vi "ScenarioScript.vi"(0 "Control In":T1) -> (1 "Control Out":T1, 2 "String":string)   [LabVIEW 2013]
uses:
  <vilib>/imath/engines/lvmath/Plug In/_Char/NIMS_CH_character datatype.ctl
  Global.vi
  <vilib>/imath/engines/lvmath2/RunTimeEngine/ErrorHandling/NIMS_Finalize Error.vi
  <vilib>/imath/engines/lvmath2/RunTimeEngine/Managers/WorkSpace/UID Generator.vi
  <vilib>/imath/engines/lvmath2/RunTimeEngine/RunTimeType/NIMS_RunTimeType_From StrictType (excl LVString).vi
  <instcachedir>/0/NIMS_RunTimeType_From StrictType (excl LVString)_4DEE718D6EB74582AA20236969C084FC.lvgen/NIMS_RunTimeType_From StrictType (excl LVString)_4DEE718D6EB74582AA20236969C084FC_033.vi
  <instcachedir>/0/NIMS_RunTimeType_From StrictType (excl LVString)_4DEE718D6EB74582AA20236969C084FC.lvgen/NIMS_RunTimeType_From StrictType (excl LVString)_4DEE718D6EB74582AA20236969C084FC_013.vi
  <instcachedir>/0/NIMS_RunTimeType_From StrictType (excl LVString)_4DEE718D6EB74582AA20236969C084FC.lvgen/NIMS_RunTimeType_From StrictType (excl LVString)_4DEE718D6EB74582AA20236969C084FC_010.vi
  <instcachedir>/0/NIMS_RunTimeType_From StrictType (excl LVString)_4DEE718D6EB74582AA20236969C084FC.lvgen/NIMS_RunTimeType_From StrictType (excl LVString)_4DEE718D6EB74582AA20236969C084FC_031.vi
  <instcachedir>/0/NIMS_RunTimeType_From StrictType (excl LVString)_4DEE718D6EB74582AA20236969C084FC.lvgen/NIMS_RunTimeType_From StrictType (excl LVString)_4DEE718D6EB74582AA20236969C084FC_008.vi
  <instcachedir>/0/NIMS_RunTimeType_From StrictType (excl LVString)_4DEE718D6EB74582AA20236969C084FC.lvgen/NIMS_RunTimeType_From StrictType (excl LVString)_4DEE718D6EB74582AA20236969C084FC_032.vi
  <vilib>/imath/engines/lvmath2/RunTimeEngine/Struct/NIMS_StructSetField.vi
  <vilib>/imath/engines/lvmath2/RunTimeEngine/Managers/SymbolTable/Clear UID.vi
  <vilib>/imath/engines/lvmath2/RunTimeEngine/Struct/NIMS_StructGetField.vi
  <vilib>/imath/engines/lvmath2/RunTimeEngine/RunTimeType/NIMS_RunTimeType_To Numeric.vi
  <instcachedir>/0/NIMS_RunTimeType_To Numeric_4795FB10E831402FABFA341B47E20681.lvgen/NIMS_RunTimeType_To Numeric_4795FB10E831402FABFA341B47E20681_011.vi
  <instcachedir>/0/NIMS_RunTimeType_To Numeric_4795FB10E831402FABFA341B47E20681.lvgen/NIMS_RunTimeType_To Numeric_4795FB10E831402FABFA341B47E20681_006.vi
  <instcachedir>/0/NIMS_RunTimeType_To Numeric_4795FB10E831402FABFA341B47E20681.lvgen/NIMS_RunTimeType_To Numeric_4795FB10E831402FABFA341B47E20681_004.vi
  <instcachedir>/0/NIMS_RunTimeType_To Numeric_4795FB10E831402FABFA341B47E20681.lvgen/NIMS_RunTimeType_To Numeric_4795FB10E831402FABFA341B47E20681_008.vi
  <instcachedir>/0/NIMS_RunTimeType_To Numeric_4795FB10E831402FABFA341B47E20681.lvgen/NIMS_RunTimeType_To Numeric_4795FB10E831402FABFA341B47E20681_010.vi
  <instcachedir>/0/NIMS_RunTimeType_To Numeric_4795FB10E831402FABFA341B47E20681.lvgen/NIMS_RunTimeType_To Numeric_4795FB10E831402FABFA341B47E20681_009.vi
  <vilib>/imath/engines/lvmath2/RunTimeEngine/NodeEndStatement/NIMS_NodeEndStatement_Output.vi
  <instcachedir>/0/NIMS_NodeEndStatement_Output_53EC0D466D134D7ABD903AC30B43404B.lvgen/NIMS_NodeEndStatement_Output_53EC0D466D134D7ABD903AC30B43404B_016.vi
  <instcachedir>/0/NIMS_NodeEndStatement_Output_53EC0D466D134D7ABD903AC30B43404B.lvgen/NIMS_NodeEndStatement_Output_53EC0D466D134D7ABD903AC30B43404B_015.vi
  <instcachedir>/0/NIMS_NodeEndStatement_Output_53EC0D466D134D7ABD903AC30B43404B.lvgen/NIMS_NodeEndStatement_Output_53EC0D466D134D7ABD903AC30B43404B_010.vi
  <vilib>/imath/engines/lvmath/Plug In/_Char/NIMS_CH_Character RV to String.vi
  <instcachedir>/0/NIMS_NodeEndStatement_Output_53EC0D466D134D7ABD903AC30B43404B.lvgen/NIMS_NodeEndStatement_Output_53EC0D466D134D7ABD903AC30B43404B_008.vi
  <instcachedir>/0/NIMS_RunTimeType_From StrictType (excl LVString)_4DEE718D6EB74582AA20236969C084FC.lvgen/NIMS_RunTimeType_From StrictType (excl LVString)_4DEE718D6EB74582AA20236969C084FC_009.vi
  <vilib>/imath/engines/lvmath2/RunTimeEngine/IndexRead/NIMS V(S).vi
  <instcachedir>/0/NIMS V(S)_0488751826AF41519A22953C041130DC.lvgen/NIMS V(S)_0488751826AF41519A22953C041130DC_000.vi
  <vilib>/imathl/engines/lvmath/Functions/Error Handling/Create Error.vi
  <vilib>/imath/engines/lvmath2/RunTimeEngine/BuiltInFunctions/sprintf/NIMS_sprintf(Str,RM).vi
  <vilib>/imath/engines/lvmath/Plug In/_Char/NIMS_CH_String to Character Array.vi
  <instcachedir>/0/NIMS_RunTimeType_From StrictType (excl LVString)_4DEE718D6EB74582AA20236969C084FC.lvgen/NIMS_RunTimeType_From StrictType (excl LVString)_4DEE718D6EB74582AA20236969C084FC_001.vi
  <vilib>/imath/engines/lvmath2/RunTimeEngine/LocalVariableDefStatement/MC_LocalVariableDefStatement_Display.vi
  <instcachedir>/0/NIMS V(S)_0488751826AF41519A22953C041130DC.lvgen/NIMS V(S)_0488751826AF41519A22953C041130DC_002.vi
  <instcachedir>/0/NIMS_RunTimeType_To Numeric_4795FB10E831402FABFA341B47E20681.lvgen/NIMS_RunTimeType_To Numeric_4795FB10E831402FABFA341B47E20681_003.vi
  <vilib>/imath/engines/lvmath2/RunTimeEngine/IndexReplace/NIMS V(S)=S.vi
  <instcachedir>/0/NIMS V(S)=S_66A18068148B4981A312229A93EA5C06.lvgen/NIMS V(S)=S_66A18068148B4981A312229A93EA5C06_000.vi
  <vilib>/imath/engines/lvmath2/RunTimeEngine/ErrorHandling/NIMS_Create Error From Enums.vi
  <instcachedir>/0/NIMS_NodeEndStatement_Output_53EC0D466D134D7ABD903AC30B43404B.lvgen/NIMS_NodeEndStatement_Output_53EC0D466D134D7ABD903AC30B43404B_001.vi
  <instcachedir>/0/NIMS V(S)_0488751826AF41519A22953C041130DC.lvgen/NIMS V(S)_0488751826AF41519A22953C041130DC_001.vi
  <vilib>/imath/engines/lvmath2/RunTimeEngine/IndexRead/NIMS M(S,S).vi
  <instcachedir>/0/NIMS M(S,S)_AC51E74150A542F7991B9634C66F3096.lvgen/NIMS M(S,S)_AC51E74150A542F7991B9634C66F3096_000.vi
  <instcachedir>/0/NIMS_NodeEndStatement_Output_53EC0D466D134D7ABD903AC30B43404B.lvgen/NIMS_NodeEndStatement_Output_53EC0D466D134D7ABD903AC30B43404B_011.vi
  <instcachedir>/0/NIMS V(S)=S_66A18068148B4981A312229A93EA5C06.lvgen/NIMS V(S)=S_66A18068148B4981A312229A93EA5C06_004.vi
  <vilib>/imath/engines/lvmath2/RunTimeEngine/BuiltInFunctions/abs/NIMS_abs(signed).vi
  <instcachedir>/0/NIMS_abs(signed)_C4FCB8E6058B49B797C7C8D53CA5F6EC.lvgen/NIMS_abs(signed)_C4FCB8E6058B49B797C7C8D53CA5F6EC_007.vi
  <instcachedir>/0/NIMS_RunTimeType_From StrictType (excl LVString)_4DEE718D6EB74582AA20236969C084FC.lvgen/NIMS_RunTimeType_From StrictType (excl LVString)_4DEE718D6EB74582AA20236969C084FC_000.vi
  <vilib>/imath/engines/lvmath2/RunTimeEngine/BuiltInFunctions/sprintf/NIMS_sprintf(Str,RS,RS).vi
  <vilib>/imath/engines/lvmath2/RunTimeEngine/BuiltInFunctions/length/NIMS_length(GV).vi
  <instcachedir>/0/NIMS_length(GV)_08A3D13377FD4E4B96F5795FBF3698FA.lvgen/NIMS_length(GV)_08A3D13377FD4E4B96F5795FBF3698FA_002.vi
  <vilib>/imath/engines/lvmath2/RunTimeEngine/BuiltInFunctions/zeros/NIMS_M=zeros(I32).vi
  <vilib>/imath/engines/lvmath2/RunTimeEngine/IndexReplace/NIMS M(S)=S.vi
  <instcachedir>/0/NIMS M(S)=S_4E994C4915F64874B0A495BA8935E304.lvgen/NIMS M(S)=S_4E994C4915F64874B0A495BA8935E304_001.vi
  <vilib>/imath/engines/lvmath2/RunTimeEngine/IndexRead/NIMS M(S).vi
  <instcachedir>/0/NIMS M(S)_B826C018497E4940AE96BD27B540B6FB.lvgen/NIMS M(S)_B826C018497E4940AE96BD27B540B6FB_000.vi
  <vilib>/imath/engines/lvmath2/RunTimeEngine/ArithmeticOperatorToken/NIMS_ArithmeticOperator_rightdiv.vi
  <instcachedir>/0/NIMS_ArithmeticOperator_rightdiv_C75411BD8BC84A93B6F1C8DA359A92EC.lvgen/NIMS_ArithmeticOperator_rightdiv_C75411BD8BC84A93B6F1C8DA359A92EC_000.vi
  <instcachedir>/0/NIMS V(S)=S_66A18068148B4981A312229A93EA5C06.lvgen/NIMS V(S)=S_66A18068148B4981A312229A93EA5C06_003.vi
  <vilib>/imath/engines/lvmath2/RunTimeEngine/CommandStatement/NIMS_CommandStatement_MaskErr.vi
  <vilib>/imath/engines/lvmath2/RunTimeEngine/BuiltInFunctions/sort/NIMS_[2o]_sort(RRowV,I32,Str).vi
  <instcachedir>/0/NIMS_[2o]_sort(RRowV,I32,Str)_CECB39279CEE49FE825BA66045B0C5B3.lvgen/NIMS_[2o]_sort(RRowV,I32,Str)_CECB39279CEE49FE825BA66045B0C5B3_000.vi
  <instcachedir>/0/NIMS_length(GV)_08A3D13377FD4E4B96F5795FBF3698FA.lvgen/NIMS_length(GV)_08A3D13377FD4E4B96F5795FBF3698FA_000.vi
  <vilib>/imath/engines/lvmath2/RunTimeEngine/CommandStatement/MC_CommandStatement_break.vi
  <vilib>/imath/engines/lvmath2/RunTimeEngine/BuiltInFunctions/findnz/NIMS_[1o]_findnz(GRowV).vi
  <instcachedir>/0/NIMS_[1o]_findnz(GRowV)_A907680C39E74AF18CBD76E991AC1137.lvgen/NIMS_[1o]_findnz(GRowV)_A907680C39E74AF18CBD76E991AC1137_001.vi
  <vilib>/imath/engines/lvmath2/RunTimeEngine/BuiltInFunctions/is_empty/NIMS_is_empty(GV).vi
  <instcachedir>/0/NIMS_is_empty(GV)_FC7E7C3D9544432CB6AA2416ADCF6D56.lvgen/NIMS_is_empty(GV)_FC7E7C3D9544432CB6AA2416ADCF6D56_000.vi
  <vilib>/imath/engines/lvmath2/RunTimeEngine/RowToken/NIMS_RowToken_M_SorRV.vi
  <instcachedir>/0/NIMS_RowToken_M_SorRV_6464340A296F47B6970F468C8541F43A.lvgen/NIMS_RowToken_M_SorRV_6464340A296F47B6970F468C8541F43A_001.vi
  <instcachedir>/0/NIMS M(S)_B826C018497E4940AE96BD27B540B6FB.lvgen/NIMS M(S)_B826C018497E4940AE96BD27B540B6FB_005.vi
  <vilib>/imath/engines/lvmath2/RunTimeEngine/BuiltInFunctions/rem/NIMS_rem_no checks.vi
  <instcachedir>/0/NIMS_rem_no checks_7935C26835844EFC868069820ED089DA.lvgen/NIMS_rem_no checks_7935C26835844EFC868069820ED089DA_008.vi
  <vilib>/imath/engines/lvmath2/RunTimeEngine/Managers/SymbolTable/NIMS_WorkSpace.lvlib
panel:
  out "SetMasterID":i32
  out "LapCounter":i32
  out "diference":dbl
  out "SlaveDistance":dbl
  out "MasterDistance":dbl
  out "Positioned":bool
  out "FirstTime":bool
  out "MasterID":i32
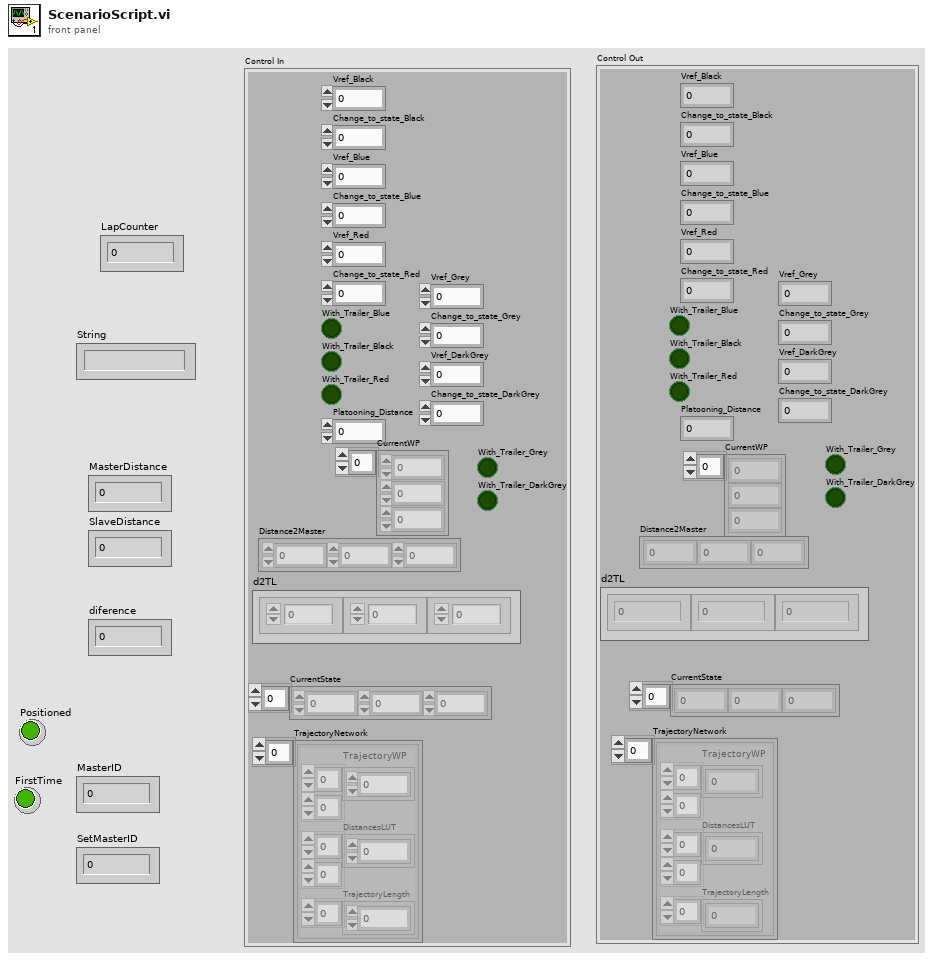
[diagram p1: front panel]
types:
  T1 = cluster{"Vref_Black":dbl, "Change_to_state_Black":i32, "Vref_Blue":dbl, "Change_to_state_Blue":i32, "Vref_Red":dbl, "Change_to_state_Red":i32, "Vref_Grey":dbl, "Change_to_state_Grey":i32, "Vref_DarkGrey":dbl, "Change_to_state_DarkGrey":i32, "With_Trailer_Blue":bool, "With_Trailer_Black":bool, "With_Trailer_Red":bool, "With_Trailer_Grey":bool, "With_Trailer_DarkGrey":bool, "Platooning_Distance":dbl, "CurrentWP":i32[], "Distance2Master":dbl[], "d2TL":dbl[], "CurrentState":i32[], "TrajectoryNetwork":cluster{"TrajectoryWP":dbl[][], "DistancesLUT":dbl[][], "TrajectoryLength":i32[]}[]}
  T2 = cluster{"TrajectoryWP":dbl[][], "DistancesLUT":dbl[][], "TrajectoryLength":i32[]}
  T3 = typedef "NIMS_CH_character datatype.ctl" = cluster{"Numeric":u8}
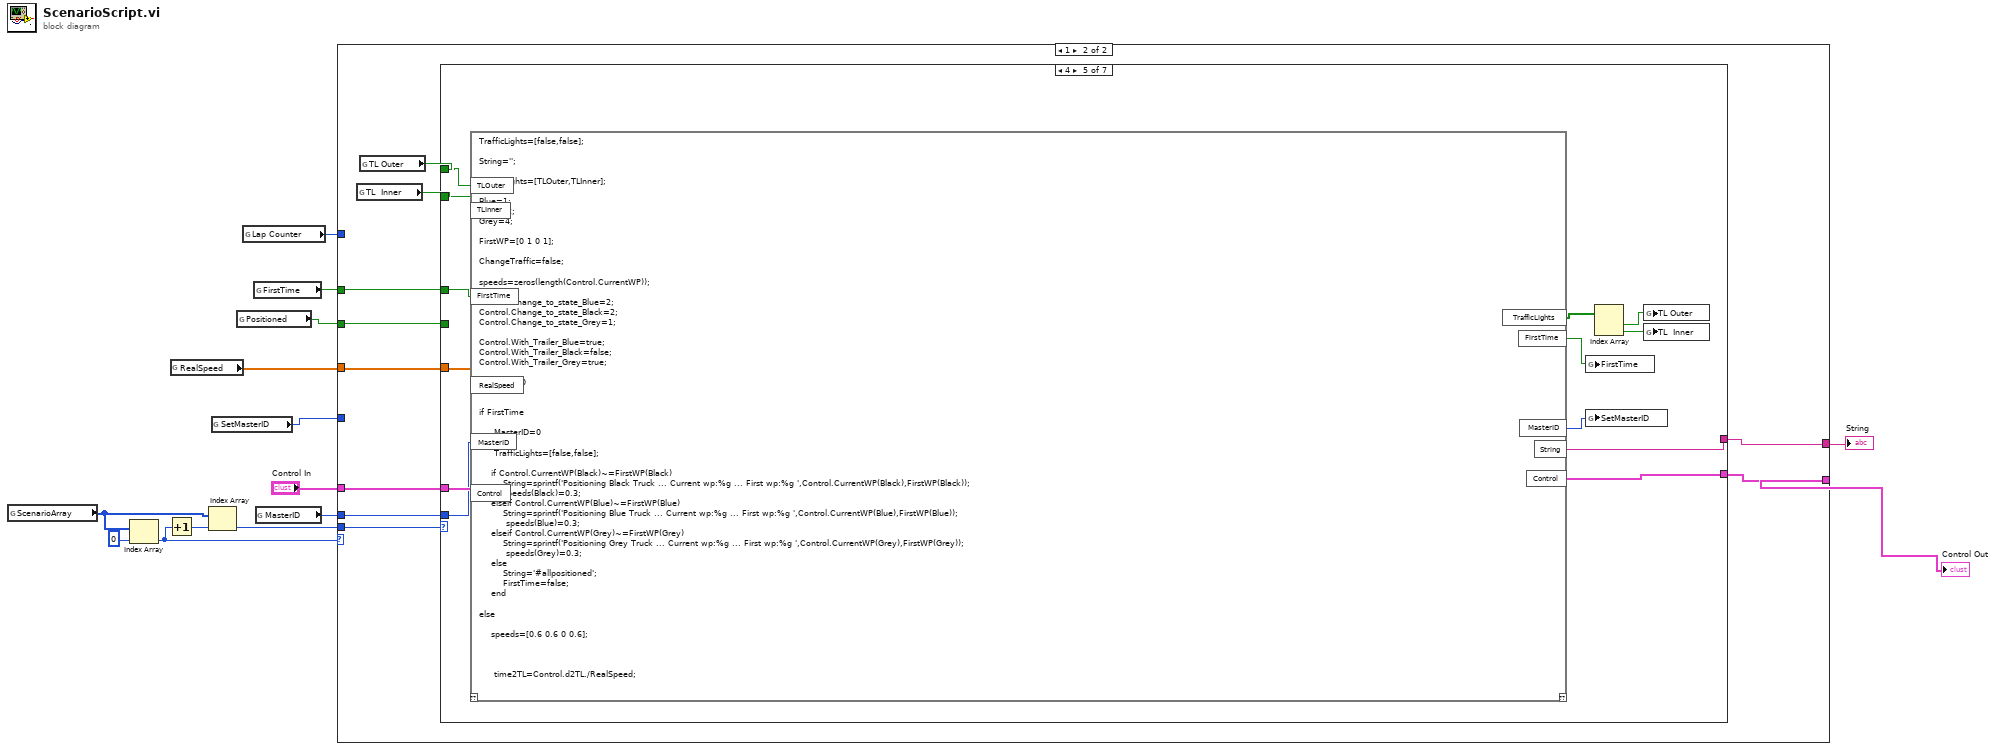
[diagram p0: block diagram]
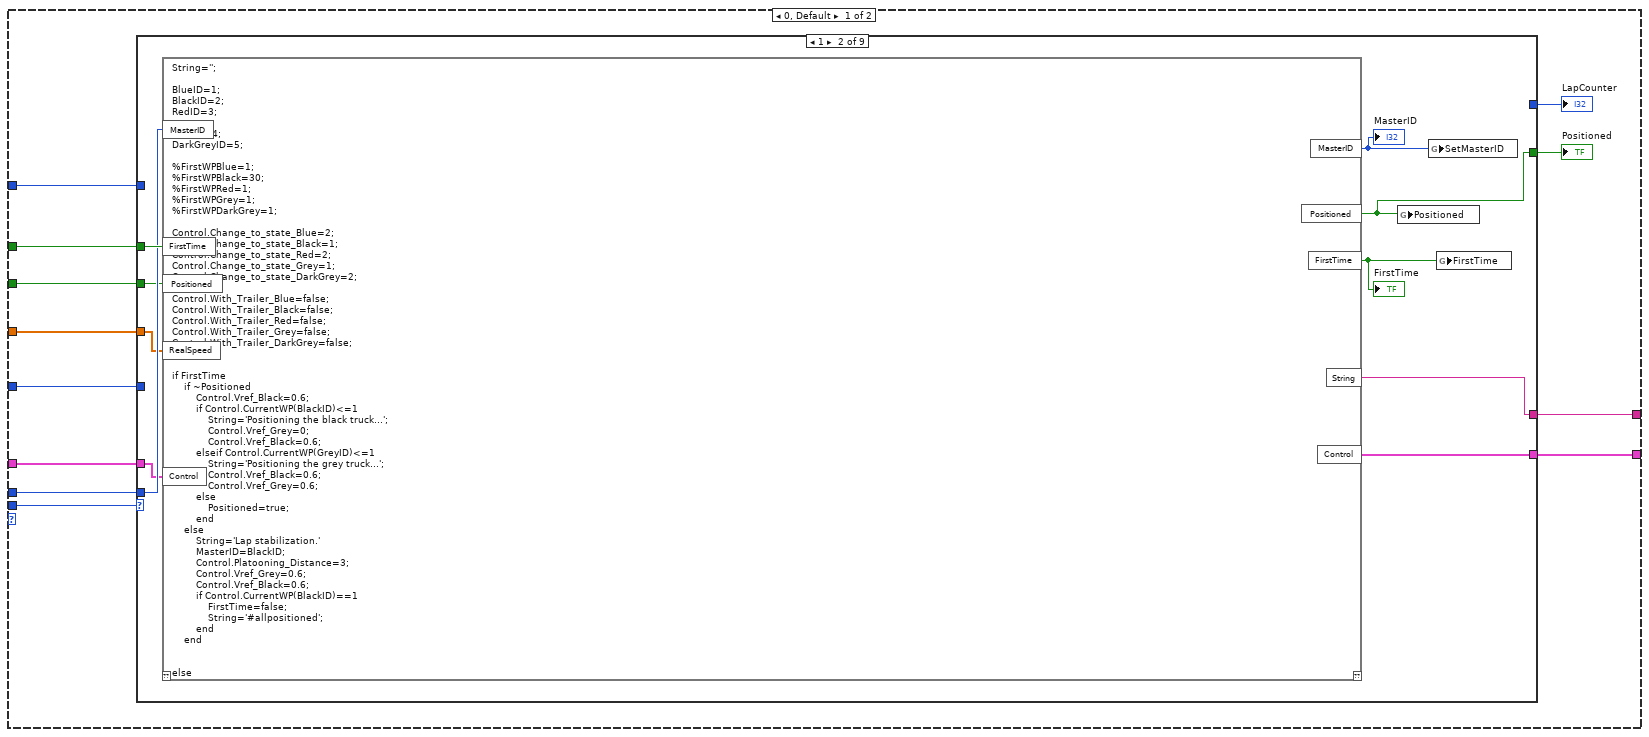
[diagram p2: hidden frame]
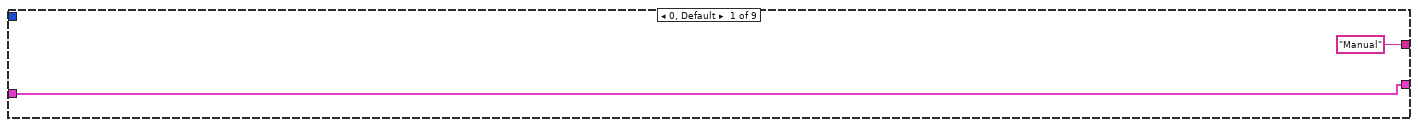
[diagram p3: hidden frame]
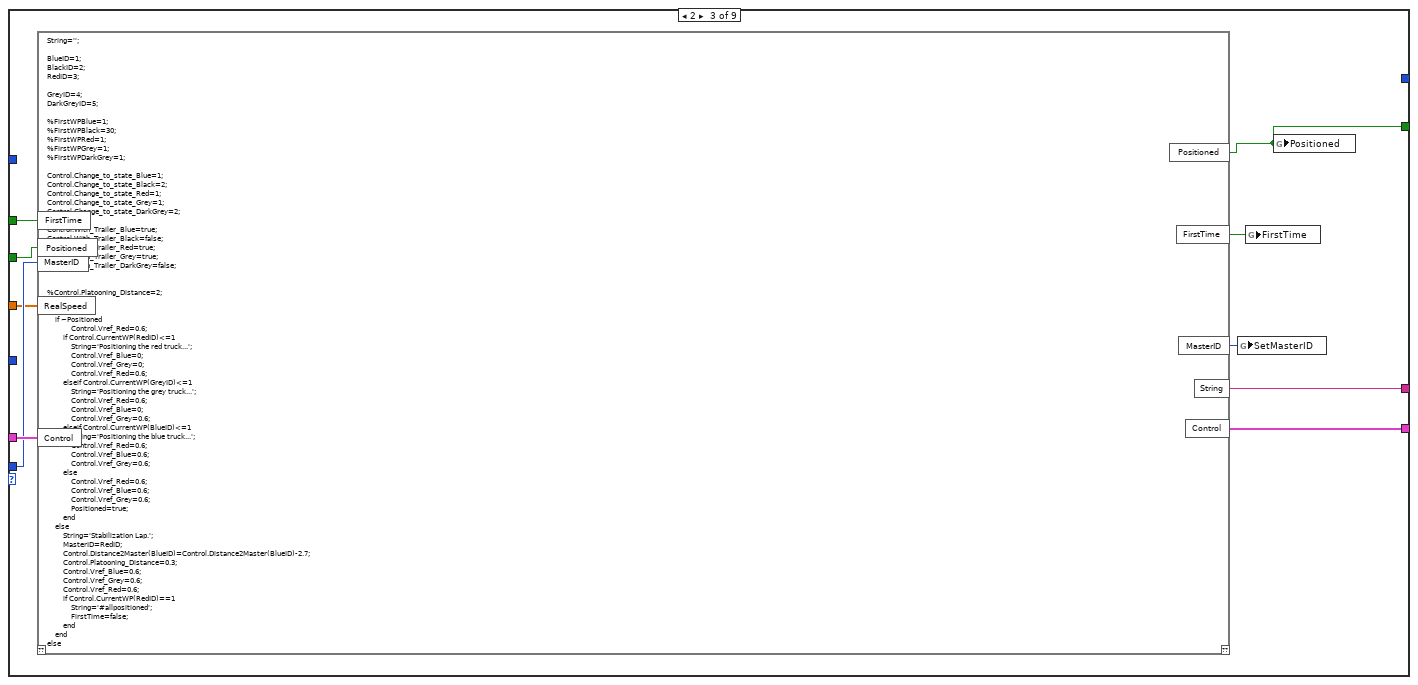
[diagram p4: hidden frame]
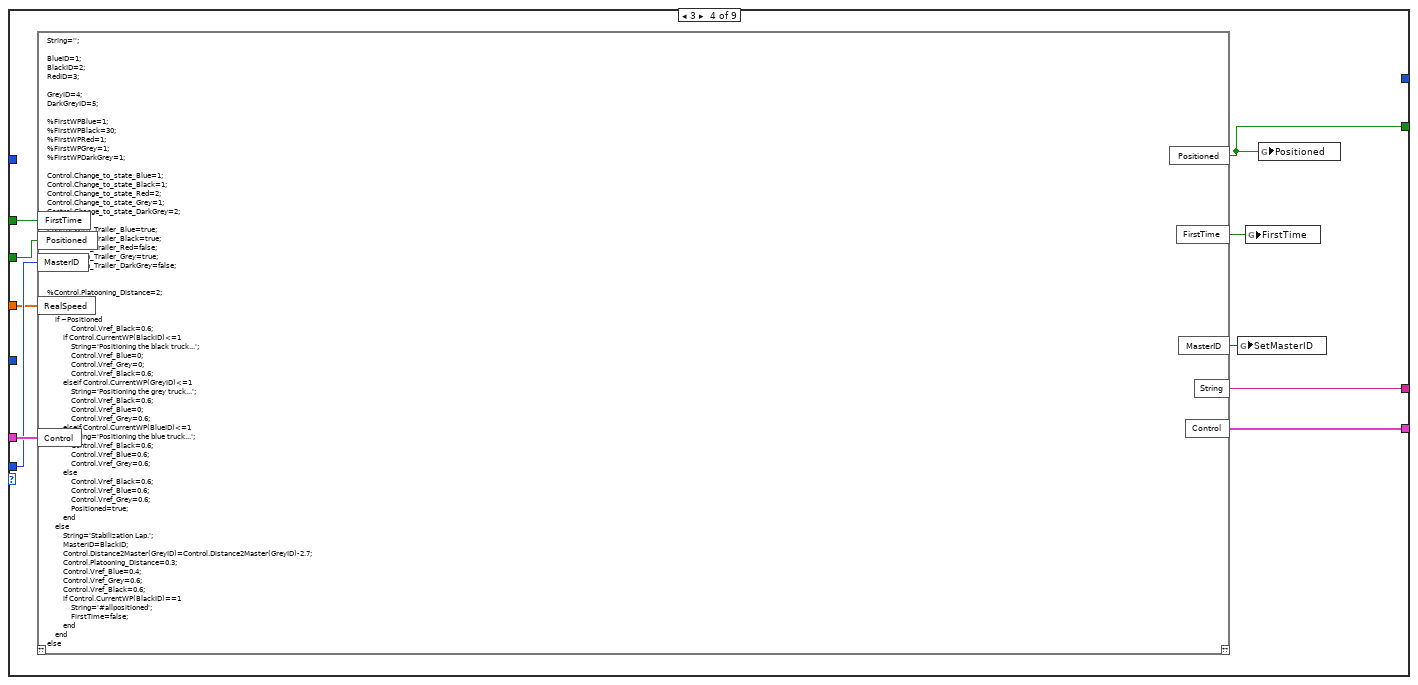
[diagram p5: hidden frame]
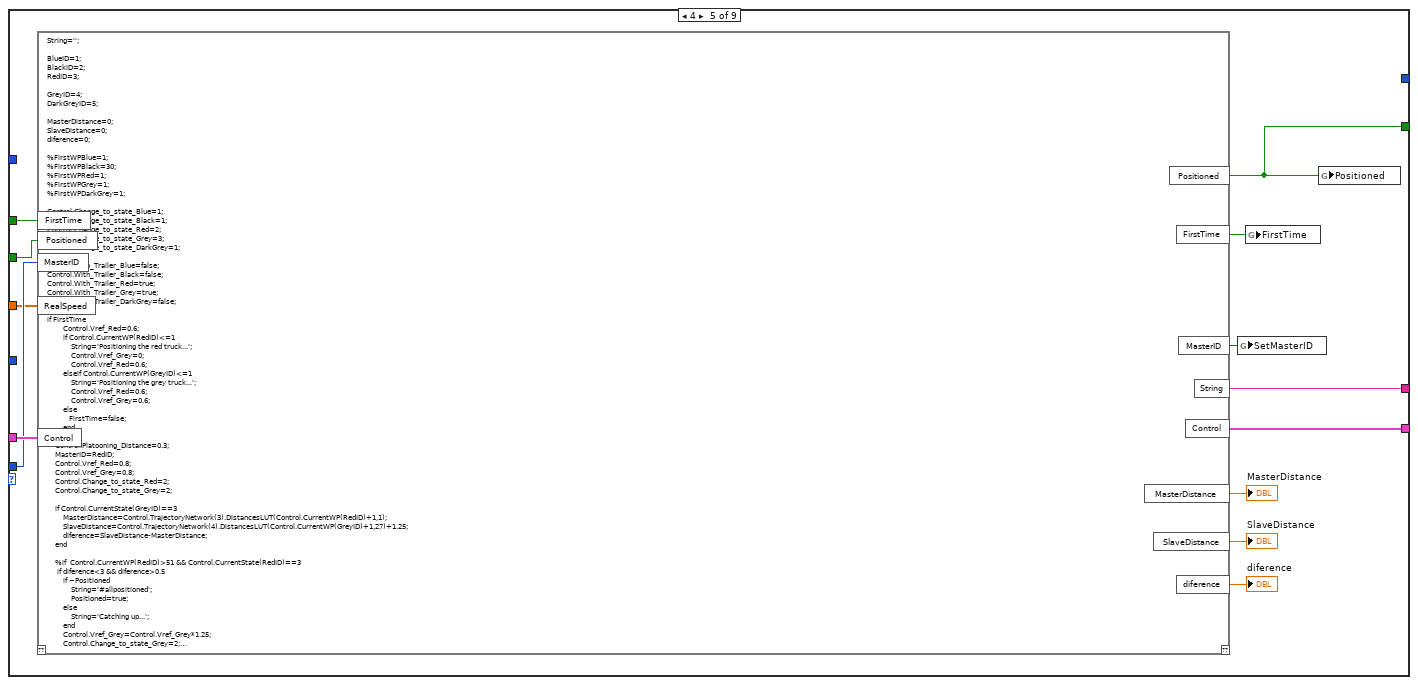
[diagram p6: hidden frame]
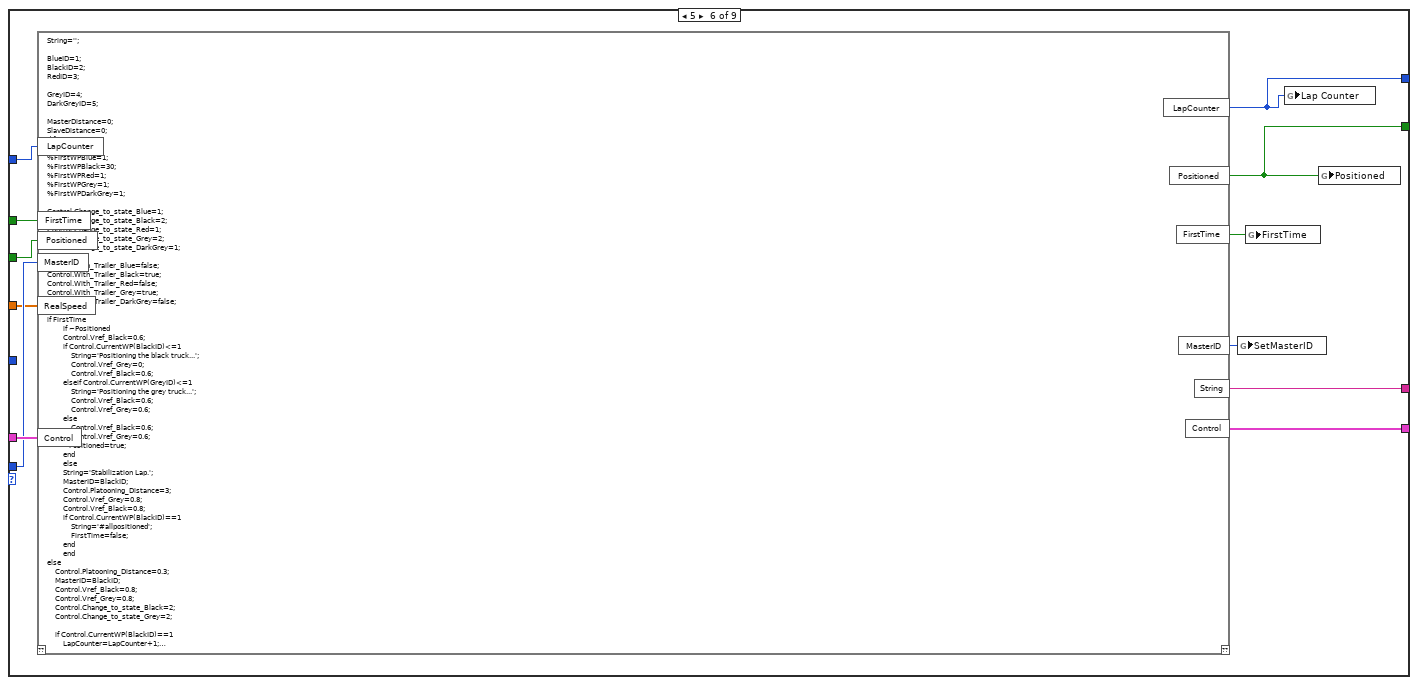
[diagram p7: hidden frame]
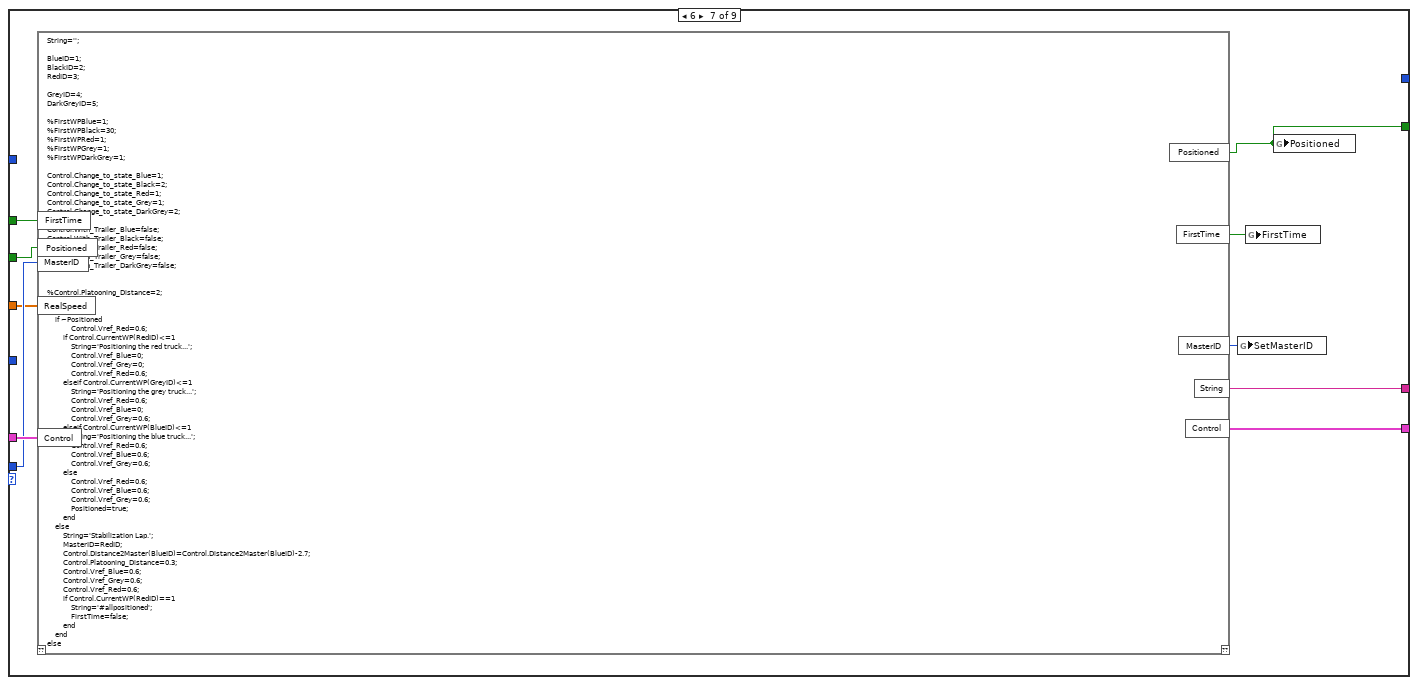
[diagram p8: hidden frame]
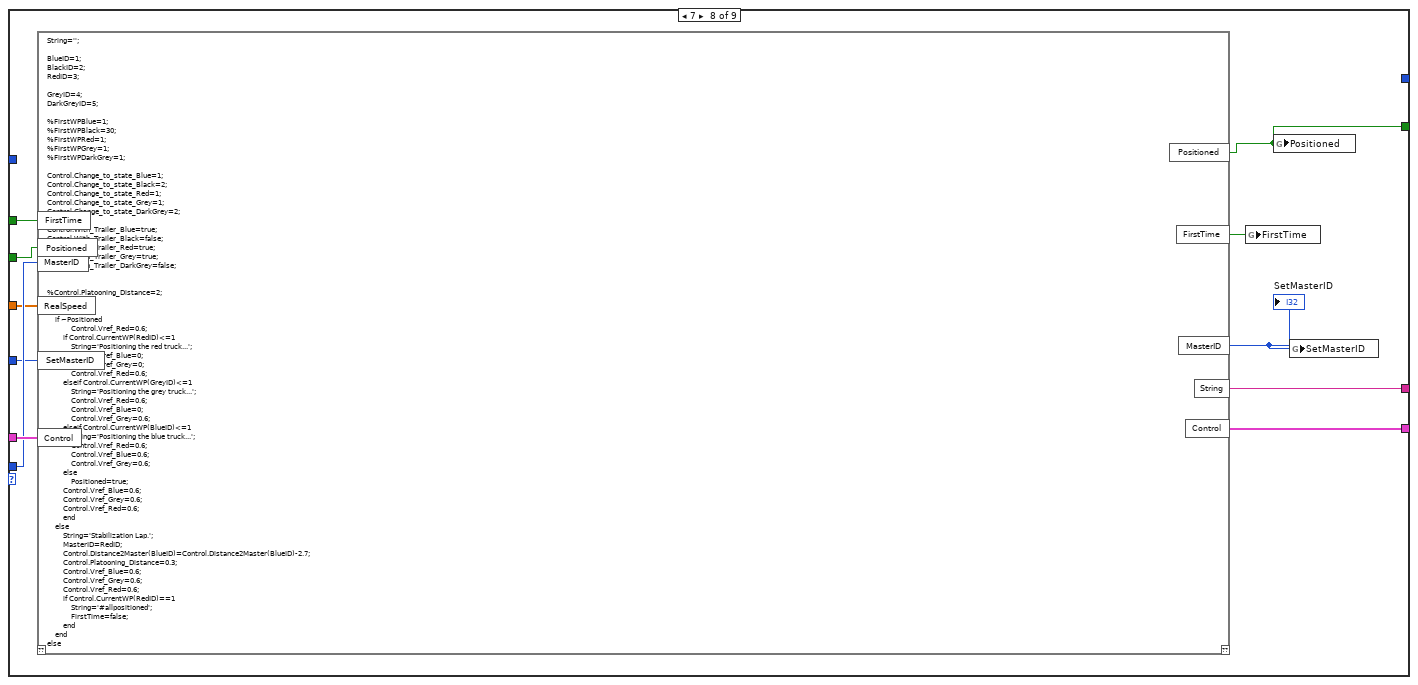
[diagram p9: hidden frame]
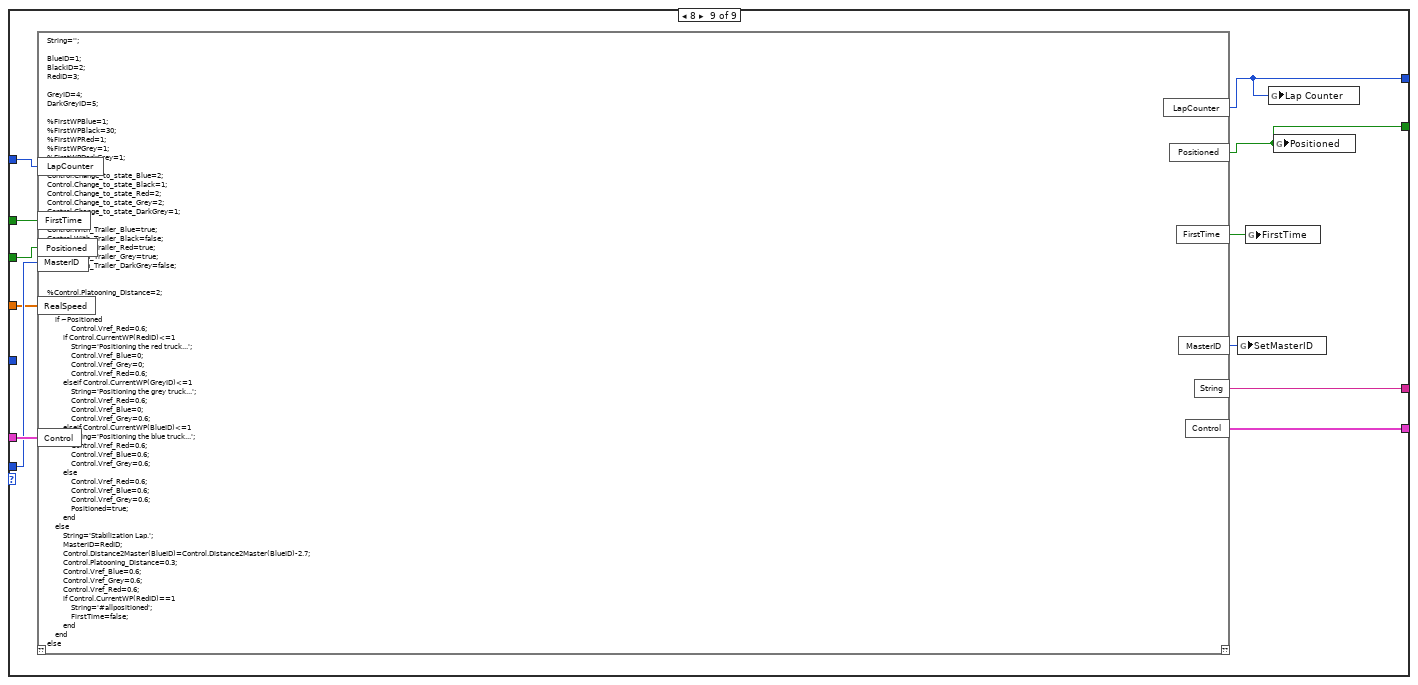
[diagram p10: hidden frame]
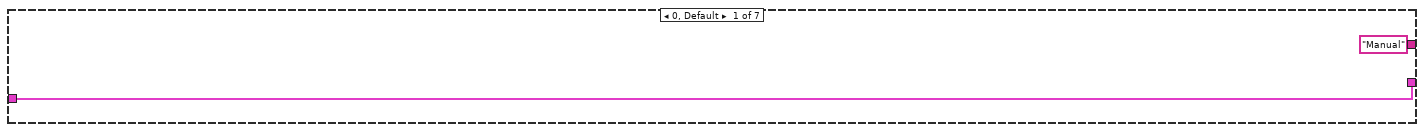
[diagram p11: hidden frame]
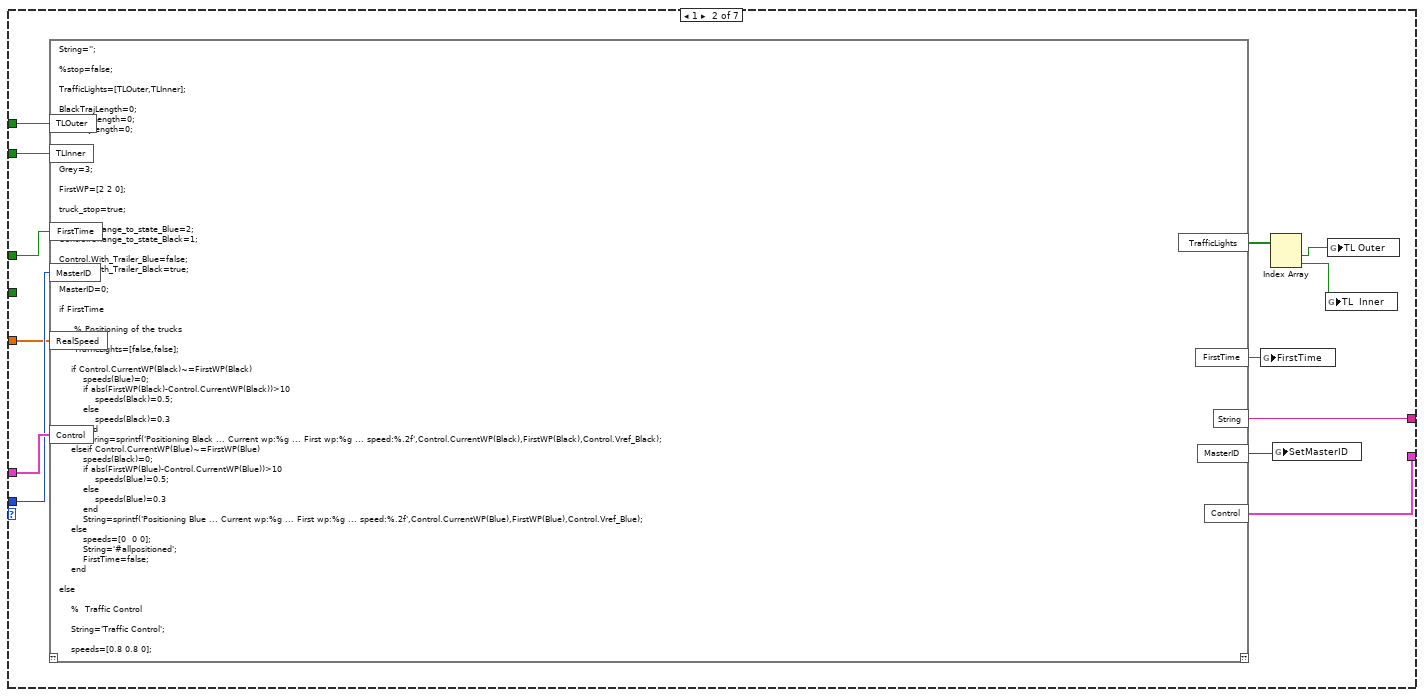
[diagram p12: hidden frame]
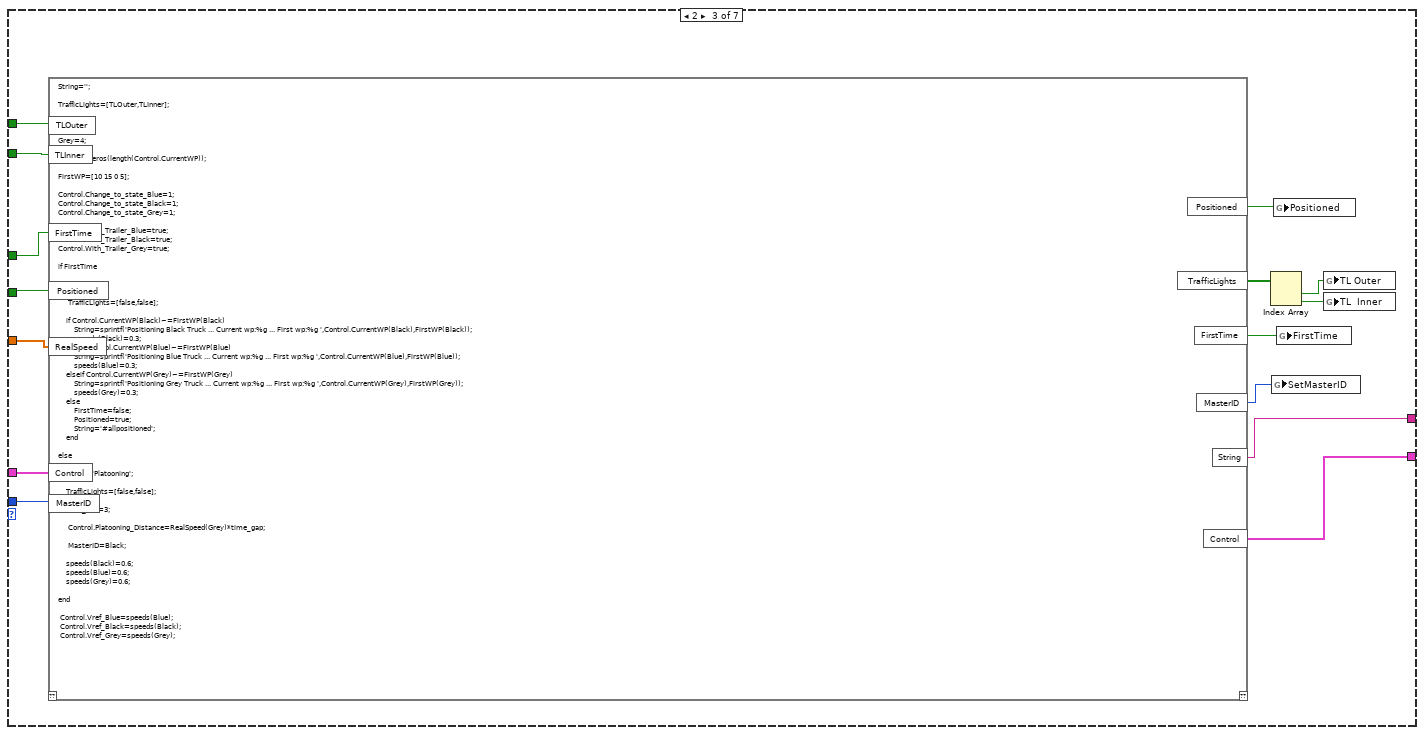
[diagram p13: hidden frame]
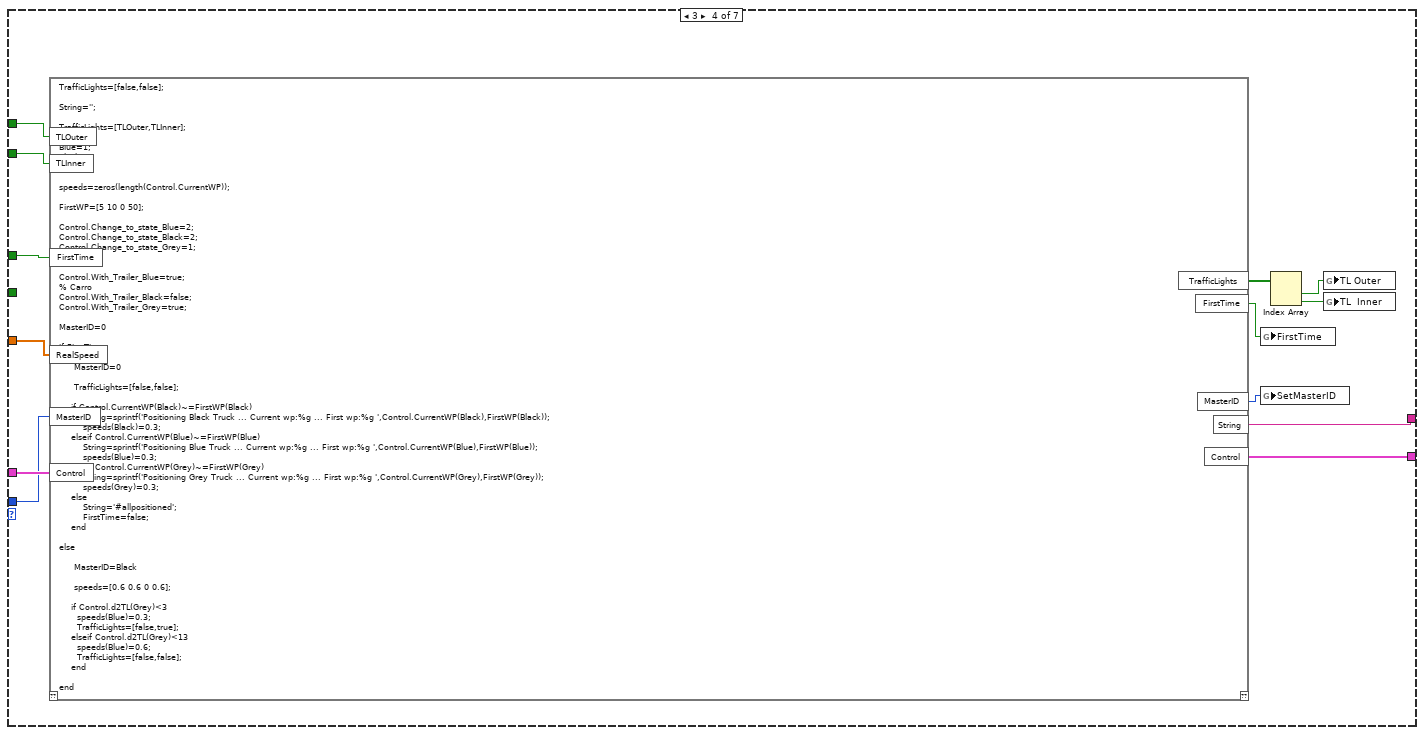
[diagram p14: hidden frame]
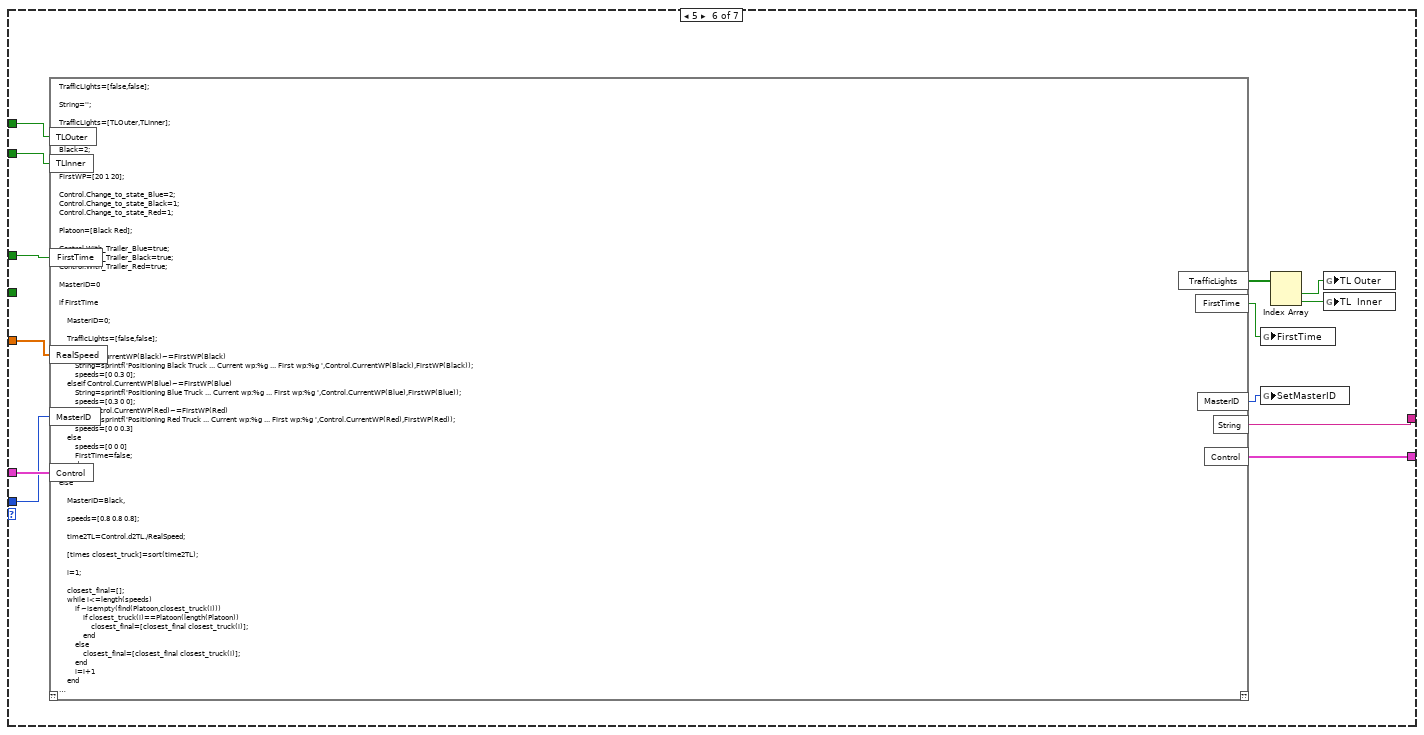
[diagram p15: hidden frame]
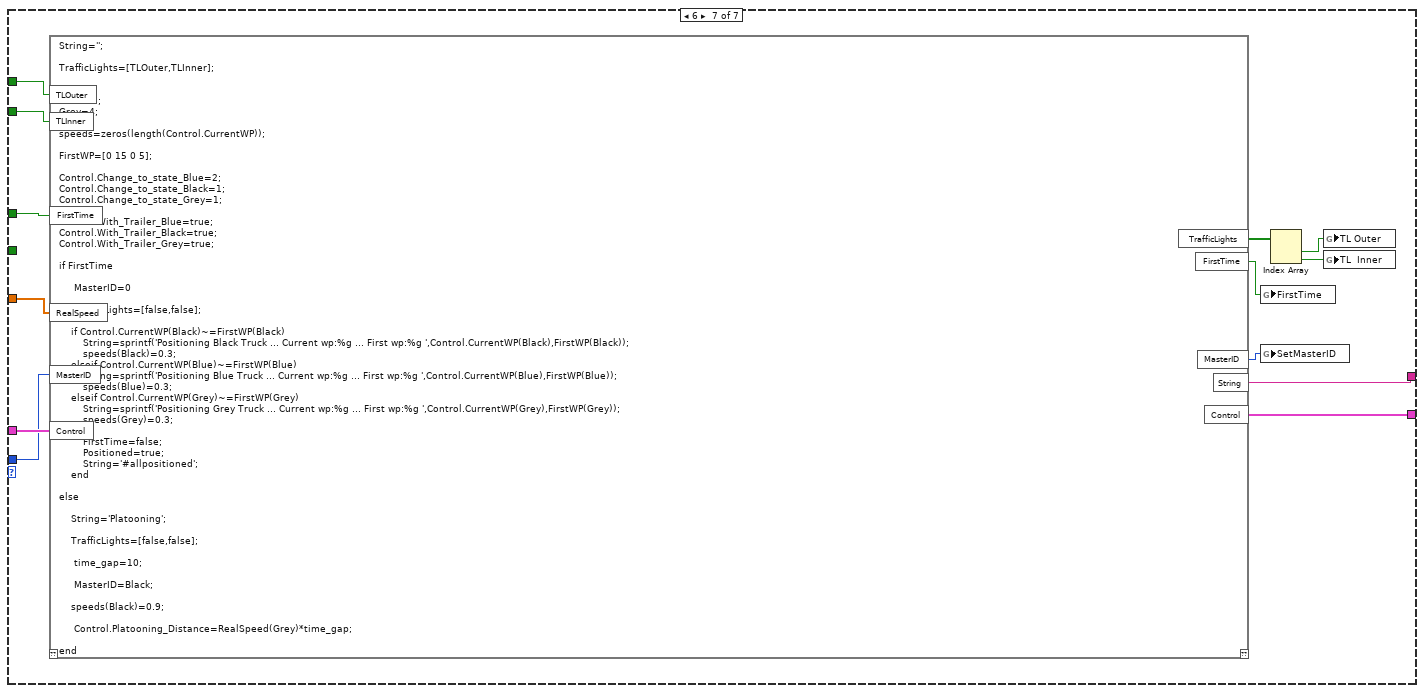
[diagram p16: hidden frame]
diagram:
  n1 = global read "Global.vi" "ScenarioArray"() -> (w13:u32[])
  n2 = Index Array(array=w13, index=0) -> (element=w12:u32)
  n3 = Increment(x=w12) -> (x+1=w11:u32)
  n4 = global read "Global.vi" "RealSpeed"() -> (w7:dbl[])
  n5 = Index Array(array=w13, index=w11) -> (element=w10:u32)
  n6 = global read "Global.vi" "SetMasterID"() -> (w1:i32)
  n7 = global read "Global.vi" "Positioned"() -> (w4:bool)
  n8 = global read "Global.vi" "Lap Counter"() -> (w2:i32)
  n9 = global read "Global.vi" "FirstTime"() -> (w9:bool)
  n10 = global read "Global.vi" "MasterID"() -> (w8:i32)
  n11 = case shown="1" w12 {
    tunnel: w10 -> [w26 w9910]
    tunnel: [w25 w9909] -> w3
    tunnel: w9 -> [w24 w9908]
    tunnel: w8 -> [w23 w9906]
    tunnel: w7 -> [w22 w9905]
    tunnel: "Control In" -> [w21 w9907]
    tunnel: [w20 w9902] -> w5
    tunnel: w4 -> [w19 w9901]
    tunnel: w2 -> [w17 _]
    tunnel: w1 -> [w15 _]
    frame 0, Default {
      n12 = case shown="1" w26 {
        tunnel: [w28 w38 w864 w2135 w3409 w4553 w5568 w6840 w8538] -> w25
        tunnel: w24 -> [_ w37 w861 w2132 w3406 w4550 w5565 w6837 w8535]
        tunnel: w23 -> [_ w35 w860 w2131 w3405 w4549 w5564 w6836 w8534]
        tunnel: w22 -> [_ w33 w859 w2130 w3404 w4548 w5563 w6835 w8533]
        tunnel: w21 -> [w28 w32 w862 w2133 w3407 w4551 w5566 w6838 w8536]
        tunnel: ["Manual" ("String") w31 w857 w2128 w3402 w4546 w5561 w6833 w8531] -> w20
        tunnel: w19 -> [_ w30 w856 w2127 w3401 w4545 w5560 w6832 w8530]
        tunnel: [_ w29 w855 w2126 w3400 w4544 w5559 w6831 w8529] -> w18
        tunnel: w17 -> [_ _ _ _ _ w4543 _ _ w8528]
        tunnel: [_ _ _ _ _ w4542 _ _ w8527] -> w16
        tunnel: w15 -> [_ _ _ _ _ _ _ w6830 _]
        frame 0, Default {
        }
        frame 1 {
          n13 = mathscript code="String='';\n\nBlueID=1;\nBlackID=2;\nRedID=3;\n\nGreyID=4;\nDarkGreyID=5;\n\n%FirstWPBlue=1;\n%FirstWPBlack=30;\n%FirstWPRed=1;\n%FirstWPGrey=1;\n%FirstWPDarkGrey=1;\n\nControl.Change_to_state_Blue=2;\nControl.Change_to_state_Black=1;\nControl.Change_to_state_Red=2;\nControl.Change_to_state_Grey=1;\nControl.Change_to_state_DarkGrey=2;\n\nControl.With_Trailer_Blue=false;\nControl.With_Trailer_Black=false;\nControl.With_Trailer_Red=false;\nControl.With_Trailer_Grey=false;\nControl.With_Trailer_DarkGrey=false;\n\n\nif FirstTime\n    if ~Positioned\n        Control.Vref_Black=0.6;\n        if Control.CurrentWP(BlackID)<=1\n            String='Positioning the black truck...';\n            Control.Vref_Grey=0;\n            Control.Vref_Black=0.6;\n        elseif Control.CurrentWP(GreyID)<=1\n            String='Positioning the grey truck...';\n            Control.Vref_Black=0.6;\n            Control.Vref_Grey=0.6;\n        else\n            Positioned=true;\n        end\n    else\n        String='Lap stabilization.'\n        MasterID=BlackID;\n        Control.Platooning_Distance=3;\n        Control.Vref_Grey=0.6;\n        Control.Vref_Black=0.6;\n        if Control.CurrentWP(BlackID)==1\n            FirstTime=false;\n            String='#allpositioned';\n        end\n    end\n    \n    \nelse\n    \n    Control.Platooning_Distance=0.3;\n    MasterID=BlackID;\n    Control.Vref_Black=0.6;\n    Control.Vref_Red=0.6;\n    \n    if Control.Distance2Master(GreyID)>Control.Platooning_Distance-0.2 && Control.Distance2Master(GreyID)<Control.Platooning_Distance+0.2\n        String='Platooning!';\n    else\n        String=sprintf('Catching up...\\n');\n    end\n    \n    \n    \n    \nend"("FirstTime"=w37, "MasterID"=w35, "RealSpeed"=w33, "Control"=w32, "Positioned"=w30) -> ("Control"=w38:T1, "FirstTime"=w36:bool, "MasterID"=w34:i32, "String"=w31:string, "Positioned"=w29:bool)  [unwired: 1 in, 1 out]
          "MasterID" <- w34
          "FirstTime" <- w36
          n14 = global write "Global.vi" "Positioned"(w29) -> ()
          n15 = global write "Global.vi" "SetMasterID"(w34) -> ()
          n16 = global write "Global.vi" "FirstTime"(w36) -> ()
        }
        frame 2 {
          n17 = mathscript code="String='';\n\nBlueID=1;\nBlackID=2;\nRedID=3;\n\nGreyID=4;\nDarkGreyID=5;\n\n%FirstWPBlue=1;\n%FirstWPBlack=30;\n%FirstWPRed=1;\n%FirstWPGrey=1;\n%FirstWPDarkGrey=1;\n\nControl.Change_to_state_Blue=1;\nControl.Change_to_state_Black=2;\nControl.Change_to_state_Red=1;\nControl.Change_to_state_Grey=1;\nControl.Change_to_state_DarkGrey=2;\n\nControl.With_Trailer_Blue=true;\nControl.With_Trailer_Black=false;\nControl.With_Trailer_Red=true;\nControl.With_Trailer_Grey=true;\nControl.With_Trailer_DarkGrey=false;\n\n\n%Control.Platooning_Distance=2;\n\nif FirstTime\n    if ~Positioned\n            Control.Vref_Red=0.6;\n        if Control.CurrentWP(RedID)<=1\n            String='Positioning the red truck...';\n            Control.Vref_Blue=0;\n            Control.Vref_Grey=0;\n            Control.Vref_Red=0.6;\n        elseif Control.CurrentWP(GreyID)<=1\n            String='Positioning the grey truck...';\n            Control.Vref_Red=0.6;\n            Control.Vref_Blue=0;\n            Control.Vref_Grey=0.6;\n        elseif Control.CurrentWP(BlueID)<=1\n            String='Positioning the blue truck...';\n            Control.Vref_Red=0.6;\n            Control.Vref_Blue=0.6;\n            Control.Vref_Grey=0.6;\n        else\n            Control.Vref_Red=0.6;\n            Control.Vref_Blue=0.6;\n            Control.Vref_Grey=0.6;\n            Positioned=true;\n        end\n    else\n        String='Stabilization Lap.';\n        MasterID=RedID;\n        Control.Distance2Master(BlueID)=Control.Distance2Master(BlueID)-2.7;\n        Control.Platooning_Distance=0.3;\n        Control.Vref_Blue=0.6;\n        Control.Vref_Grey=0.6;\n        Control.Vref_Red=0.6;\n        if Control.CurrentWP(RedID)==1\n            String='#allpositioned';\n            FirstTime=false;\n        end\n    end\nelse\n    \n    \n    MasterID=RedID;\n    Control.Platooning_Distance=0.3;\n    Control.Vref_Blue=0.6;\n    Control.Vref_Grey=0.6;\n    Control.Vref_Red=0.6;\n    \n    if Control.Distance2Master(GreyID)>Control.Platooning_Distance-0.2 && Control.Distance2Master(GreyID)<Control.Platooning_Distance+0.2 && Control.Distance2Master(BlueID)>Control.Platooning_Distance-0.2 && Control.Distance2Master(BlueID)<Control.Platooning_Distance+0.2\n        String='The blue and grey truck are platooning!';\n    elseif Control.Distance2Master(GreyID)>Control.Platooning_Distance-0.2 && Control.Distance2Master(GreyID)<Control.Platooning_Distance+0.2\n        String='The grey truck is platooning!';\n    elseif Control.Distance2Master(BlueID)>Control.Platooning_Distance-0.2 && Control.Distance2Master(BlueID)<Control.Platooning_Distance+0.2\n        String='The blue truck is platooning!';\n    else\n        String=sprintf('Catching up...\\n');\n    end\n    \nend"("Control"=w862, "FirstTime"=w861, "MasterID"=w860, "RealSpeed"=w859, "Positioned"=w856) -> ("Control"=w864:T1, "FirstTime"=w863:bool, "MasterID"=w858:i32, "String"=w857:string, "Positioned"=w855:bool)  [unwired: 1 in, 1 out]
          n18 = global write "Global.vi" "SetMasterID"(w858) -> ()
          n19 = global write "Global.vi" "FirstTime"(w863) -> ()
          n20 = global write "Global.vi" "Positioned"(w855) -> ()
        }
        frame 3 {
          n21 = mathscript code="String='';\n\nBlueID=1;\nBlackID=2;\nRedID=3;\n\nGreyID=4;\nDarkGreyID=5;\n\n%FirstWPBlue=1;\n%FirstWPBlack=30;\n%FirstWPRed=1;\n%FirstWPGrey=1;\n%FirstWPDarkGrey=1;\n\nControl.Change_to_state_Blue=1;\nControl.Change_to_state_Black=1;\nControl.Change_to_state_Red=2;\nControl.Change_to_state_Grey=1;\nControl.Change_to_state_DarkGrey=2;\n\nControl.With_Trailer_Blue=true;\nControl.With_Trailer_Black=true;\nControl.With_Trailer_Red=false;\nControl.With_Trailer_Grey=true;\nControl.With_Trailer_DarkGrey=false;\n\n\n%Control.Platooning_Distance=2;\n\nif FirstTime\n    if ~Positioned\n            Control.Vref_Black=0.6;\n        if Control.CurrentWP(BlackID)<=1\n            String='Positioning the black truck...';\n            Control.Vref_Blue=0;\n            Control.Vref_Grey=0;\n            Control.Vref_Black=0.6;\n        elseif Control.CurrentWP(GreyID)<=1\n            String='Positioning the grey truck...';\n            Control.Vref_Black=0.6;\n            Control.Vref_Blue=0;\n            Control.Vref_Grey=0.6;\n        elseif Control.CurrentWP(BlueID)<=1\n            String='Positioning the blue truck...';\n            Control.Vref_Black=0.6;\n            Control.Vref_Blue=0.6;\n            Control.Vref_Grey=0.6;\n        else\n            Control.Vref_Black=0.6;\n            Control.Vref_Blue=0.6;\n            Control.Vref_Grey=0.6;\n            Positioned=true;\n        end\n    else\n        String='Stabilization Lap.';\n        MasterID=BlackID;\n        Control.Distance2Master(GreyID)=Control.Distance2Master(GreyID)-2.7;\n        Control.Platooning_Distance=0.3;\n        Control.Vref_Blue=0.4;\n        Control.Vref_Grey=0.6;\n        Control.Vref_Black=0.6;\n        if Control.CurrentWP(BlackID)==1\n            String='#allpositioned';\n            FirstTime=false;\n        end\n    end\nelse\n    \n    \n    MasterID=BlackID;\n    Control.Platooning_Distance=0.3;\n    Control.Vref_Blue=0.6;\n    Control.Vref_Grey=0.6;\n    Control.Vref_Black=0.6;\n    \n    if Control.Distance2Master(GreyID)>Control.Platooning_Distance-0.2 && Control.Distance2Master(GreyID)<Control.Platooning_Distance+0.2 && Control.Distance2Master(BlueID)>Control.Platooning_Distance-0.2 && Control.Distance2Master(BlueID)<Control.Platooning_Distance+0.2\n        String='The blue and grey truck are platooning!';\n    elseif Control.Distance2Master(GreyID)>Control.Platooning_Distance-0.2 && Control.Distance2Master(GreyID)<Control.Platooning_Distance+0.2\n        String='The blue truck is platooning!';\n    elseif Control.Distance2Master(BlueID)>Control.Platooning_Distance-0.2 && Control.Distance2Master(BlueID)<Control.Platooning_Distance+0.2\n        String='The grey truck is platooning!';\n    else\n        String=sprintf('Catching up...\\n');\n    end\n    \nend"("Control"=w2133, "FirstTime"=w2132, "MasterID"=w2131, "RealSpeed"=w2130, "Positioned"=w2127) -> ("Control"=w2135:T1, "FirstTime"=w2134:bool, "MasterID"=w2129:i32, "String"=w2128:string, "Positioned"=w2126:bool)  [unwired: 1 in, 1 out]
          n22 = global write "Global.vi" "SetMasterID"(w2129) -> ()
          n23 = global write "Global.vi" "FirstTime"(w2134) -> ()
          n24 = global write "Global.vi" "Positioned"(w2126) -> ()
        }
        frame 4 {
          n25 = mathscript code="String='';\n\nBlueID=1;\nBlackID=2;\nRedID=3;\n\nGreyID=4;\nDarkGreyID=5;\n\nMasterDistance=0;\nSlaveDistance=0;\ndiference=0;\n\n%FirstWPBlue=1;\n%FirstWPBlack=30;\n%FirstWPRed=1;\n%FirstWPGrey=1;\n%FirstWPDarkGrey=1;\n\nControl.Change_to_state_Blue=1;\nControl.Change_to_state_Black=1;\nControl.Change_to_state_Red=2;\nControl.Change_to_state_Grey=3;\nControl.Change_to_state_DarkGrey=1;\n\nControl.With_Trailer_Blue=false;\nControl.With_Trailer_Black=false;\nControl.With_Trailer_Red=true;\nControl.With_Trailer_Grey=true;\nControl.With_Trailer_DarkGrey=false;\n\nif FirstTime\n        Control.Vref_Red=0.6;\n        if Control.CurrentWP(RedID)<=1\n            String='Positioning the red truck...';\n            Control.Vref_Grey=0;\n            Control.Vref_Red=0.6;\n        elseif Control.CurrentWP(GreyID)<=1\n            String='Positioning the grey truck...';\n            Control.Vref_Red=0.6;\n            Control.Vref_Grey=0.6;\n        else\n           FirstTime=false;\n        end\nelse\n    Control.Platooning_Distance=0.3;\n    MasterID=RedID;\n    Control.Vref_Red=0.8;\n    Control.Vref_Grey=0.8;\n    Control.Change_to_state_Red=2;\n    Control.Change_to_state_Grey=2;\n\n    if Control.CurrentState(GreyID)==3\n        MasterDistance=Control.TrajectoryNetwork(3).DistancesLUT(Control.CurrentWP(RedID)+1,1);\n        SlaveDistance=Control.TrajectoryNetwork(4).DistancesLUT(Control.CurrentWP(GreyID)+1,27)+1.25;\n        diference=SlaveDistance-MasterDistance;\n    end\n\n    %if  Control.CurrentWP(RedID)>51 && Control.CurrentState(RedID)==3\n     if diference<3 && diference>0.5\n        if ~Positioned\n            String='#allpositioned';\n            Positioned=true;\n        else\n            String='Catching up...';\n        end\n        Control.Vref_Grey=Control.Vref_Grey*1.25;\n        Control.Change_to_state_Grey=2;\n    elseif Control.CurrentState(GreyID)==3\n        if ~Positioned\n            String='Expecting for the best time to start to catch up...';\n        end\n        Control.Change_to_state_Grey=3;\n    end\n    \n \n    \n    if Control.Distance2Master(GreyID)>Control.Platooning_Distance-0.2 && Control.Distance2Master(GreyID)<Control.Platooning_Distance+0.2\n        String='Platooning!';\n    elseif Control.CurrentState(GreyID)==Control.CurrentState(RedID)\n        String=sprintf('Catching up...\\n');\n    end\n    \nend"("Control"=w3407, "FirstTime"=w3406, "MasterID"=w3405, "RealSpeed"=w3404, "Positioned"=w3401) -> ("Control"=w3409:T1, "FirstTime"=w3408:bool, "MasterID"=w3403:i32, "String"=w3402:string, "Positioned"=w3400:bool, "MasterDistance"=→"MasterDistance":dbl, "SlaveDistance"=→"SlaveDistance":dbl, "diference"=→"diference":dbl)  [unwired: 1 in, 1 out]
          n26 = global write "Global.vi" "SetMasterID"(w3403) -> ()
          n27 = global write "Global.vi" "FirstTime"(w3408) -> ()
          n28 = global write "Global.vi" "Positioned"(w3400) -> ()
        }
        frame 5 {
          n29 = mathscript code="String='';\n\nBlueID=1;\nBlackID=2;\nRedID=3;\n\nGreyID=4;\nDarkGreyID=5;\n\nMasterDistance=0;\nSlaveDistance=0;\ndiference=0;\n\n%FirstWPBlue=1;\n%FirstWPBlack=30;\n%FirstWPRed=1;\n%FirstWPGrey=1;\n%FirstWPDarkGrey=1;\n\nControl.Change_to_state_Blue=1;\nControl.Change_to_state_Black=2;\nControl.Change_to_state_Red=1;\nControl.Change_to_state_Grey=2;\nControl.Change_to_state_DarkGrey=1;\n\nControl.With_Trailer_Blue=false;\nControl.With_Trailer_Black=true;\nControl.With_Trailer_Red=false;\nControl.With_Trailer_Grey=true;\nControl.With_Trailer_DarkGrey=false;\n\nif FirstTime\n        if ~Positioned\n        Control.Vref_Black=0.6;\n        if Control.CurrentWP(BlackID)<=1\n            String='Positioning the black truck...';\n            Control.Vref_Grey=0;\n            Control.Vref_Black=0.6;\n        elseif Control.CurrentWP(GreyID)<=1\n            String='Positioning the grey truck...';\n            Control.Vref_Black=0.6;\n            Control.Vref_Grey=0.6;\n        else\n            Control.Vref_Black=0.6;\n            Control.Vref_Grey=0.6;\n           Positioned=true;\n        end\n        else\n        String='Stabilization Lap.';\n        MasterID=BlackID;\n        Control.Platooning_Distance=3;\n        Control.Vref_Grey=0.8;\n        Control.Vref_Black=0.8;\n        if Control.CurrentWP(BlackID)==1\n            String='#allpositioned';\n            FirstTime=false;\n        end\n        end\nelse\n    Control.Platooning_Distance=0.3;\n    MasterID=BlackID;\n    Control.Vref_Black=0.8;\n    Control.Vref_Grey=0.8;\n    Control.Change_to_state_Black=2;\n    Control.Change_to_state_Grey=2;\n  \n    if Control.CurrentWP(BlackID)==1\n        LapCounter=LapCounter+1;\n    end\n\n     if LapCounter>10\n        Control.Change_to_state_Black=3;\n        string='The master exited the road. Both trucks are now alone...'\n     end \n\n    if Control.Distance2Master(GreyID)>Control.Platooning_Distance-0.2 && Control.Distance2Master(GreyID)<Control.Platooning_Distance+0.2\n        String='Platooning!';\n    elseif Control.CurrentState(GreyID)==Control.CurrentState(BlackID)\n        String=sprintf('Catching up...\\n');\n    end\n    \nend"("Control"=w4551, "FirstTime"=w4550, "MasterID"=w4549, "RealSpeed"=w4548, "Positioned"=w4545, "LapCounter"=w4543) -> ("Control"=w4553:T1, "FirstTime"=w4552:bool, "MasterID"=w4547:i32, "String"=w4546:string, "Positioned"=w4544:bool, "LapCounter"=w4542:i32)  [unwired: 1 in, 1 out]
          n30 = global write "Global.vi" "SetMasterID"(w4547) -> ()
          n31 = global write "Global.vi" "FirstTime"(w4552) -> ()
          n32 = global write "Global.vi" "Lap Counter"(w4542) -> ()
          n33 = global write "Global.vi" "Positioned"(w4544) -> ()
        }
        frame 6 {
          n34 = mathscript code="String='';\n\nBlueID=1;\nBlackID=2;\nRedID=3;\n\nGreyID=4;\nDarkGreyID=5;\n\n%FirstWPBlue=1;\n%FirstWPBlack=30;\n%FirstWPRed=1;\n%FirstWPGrey=1;\n%FirstWPDarkGrey=1;\n\nControl.Change_to_state_Blue=1;\nControl.Change_to_state_Black=2;\nControl.Change_to_state_Red=1;\nControl.Change_to_state_Grey=1;\nControl.Change_to_state_DarkGrey=2;\n\nControl.With_Trailer_Blue=false;\nControl.With_Trailer_Black=false;\nControl.With_Trailer_Red=false;\nControl.With_Trailer_Grey=false;\nControl.With_Trailer_DarkGrey=false;\n\n\n%Control.Platooning_Distance=2;\n\nif FirstTime\n    if ~Positioned\n            Control.Vref_Red=0.6;\n        if Control.CurrentWP(RedID)<=1\n            String='Positioning the red truck...';\n            Control.Vref_Blue=0;\n            Control.Vref_Grey=0;\n            Control.Vref_Red=0.6;\n        elseif Control.CurrentWP(GreyID)<=1\n            String='Positioning the grey truck...';\n            Control.Vref_Red=0.6;\n            Control.Vref_Blue=0;\n            Control.Vref_Grey=0.6;\n        elseif Control.CurrentWP(BlueID)<=1\n            String='Positioning the blue truck...';\n            Control.Vref_Red=0.6;\n            Control.Vref_Blue=0.6;\n            Control.Vref_Grey=0.6;\n        else\n            Control.Vref_Red=0.6;\n            Control.Vref_Blue=0.6;\n            Control.Vref_Grey=0.6;\n            Positioned=true;\n        end\n    else\n        String='Stabilization Lap.';\n        MasterID=RedID;\n        Control.Distance2Master(BlueID)=Control.Distance2Master(BlueID)-2.7;\n        Control.Platooning_Distance=0.3;\n        Control.Vref_Blue=0.6;\n        Control.Vref_Grey=0.6;\n        Control.Vref_Red=0.6;\n        if Control.CurrentWP(RedID)==1\n            String='#allpositioned';\n            FirstTime=false;\n        end\n    end\nelse\n    \n    \n    MasterID=RedID;\n    Control.Platooning_Distance=0.3;\n    Control.Vref_Blue=0.6;\n    Control.Vref_Grey=0.6;\n    Control.Vref_Red=0.6;\n    \n    if Control.Distance2Master(GreyID)>Control.Platooning_Distance-0.2 && Control.Distance2Master(GreyID)<Control.Platooning_Distance+0.2 && Control.Distance2Master(BlueID)>Control.Platooning_Distance-0.2 && Control.Distance2Master(BlueID)<Control.Platooning_Distance+0.2\n        String='The blue and grey truck are platooning!';\n    elseif Control.Distance2Master(GreyID)>Control.Platooning_Distance-0.2 && Control.Distance2Master(GreyID)<Control.Platooning_Distance+0.2\n        String='The grey truck is platooning!';\n    elseif Control.Distance2Master(BlueID)>Control.Platooning_Distance-0.2 && Control.Distance2Master(BlueID)<Control.Platooning_Distance+0.2\n        String='The blue truck is platooning!';\n    else\n        String=sprintf('Catching up...\\n');\n    end\n    \nend"("Control"=w5566, "FirstTime"=w5565, "MasterID"=w5564, "RealSpeed"=w5563, "Positioned"=w5560) -> ("Control"=w5568:T1, "FirstTime"=w5567:bool, "MasterID"=w5562:i32, "String"=w5561:string, "Positioned"=w5559:bool)  [unwired: 1 in, 1 out]
          n35 = global write "Global.vi" "SetMasterID"(w5562) -> ()
          n36 = global write "Global.vi" "FirstTime"(w5567) -> ()
          n37 = global write "Global.vi" "Positioned"(w5559) -> ()
        }
        frame 7 {
          n38 = mathscript code="String='';\n\nBlueID=1;\nBlackID=2;\nRedID=3;\n\nGreyID=4;\nDarkGreyID=5;\n\n%FirstWPBlue=1;\n%FirstWPBlack=30;\n%FirstWPRed=1;\n%FirstWPGrey=1;\n%FirstWPDarkGrey=1;\n\nControl.Change_to_state_Blue=1;\nControl.Change_to_state_Black=2;\nControl.Change_to_state_Red=1;\nControl.Change_to_state_Grey=1;\nControl.Change_to_state_DarkGrey=2;\n\nControl.With_Trailer_Blue=true;\nControl.With_Trailer_Black=false;\nControl.With_Trailer_Red=true;\nControl.With_Trailer_Grey=true;\nControl.With_Trailer_DarkGrey=false;\n\n\n%Control.Platooning_Distance=2;\n\nif FirstTime\n    if ~Positioned\n            Control.Vref_Red=0.6;\n        if Control.CurrentWP(RedID)<=1\n            String='Positioning the red truck...';\n            Control.Vref_Blue=0;\n            Control.Vref_Grey=0;\n            Control.Vref_Red=0.6;\n        elseif Control.CurrentWP(GreyID)<=1\n            String='Positioning the grey truck...';\n            Control.Vref_Red=0.6;\n            Control.Vref_Blue=0;\n            Control.Vref_Grey=0.6;\n        elseif Control.CurrentWP(BlueID)<=1\n            String='Positioning the blue truck...';\n            Control.Vref_Red=0.6;\n            Control.Vref_Blue=0.6;\n            Control.Vref_Grey=0.6;\n        else\n            Positioned=true;\n        Control.Vref_Blue=0.6;\n        Control.Vref_Grey=0.6;\n        Control.Vref_Red=0.6;\n        end\n    else\n        String='Stabilization Lap.';\n        MasterID=RedID;\n        Control.Distance2Master(BlueID)=Control.Distance2Master(BlueID)-2.7;\n        Control.Platooning_Distance=0.3;\n        Control.Vref_Blue=0.6;\n        Control.Vref_Grey=0.6;\n        Control.Vref_Red=0.6;\n        if Control.CurrentWP(RedID)==1\n            String='#allpositioned';\n            FirstTime=false;\n        end\n    end\nelse\n    \n    if SetMasterID==RedID\n    MasterID=RedID;\n    Control.Platooning_Distance=0.3;\n    Control.Vref_Blue=0.6;\n    Control.Vref_Grey=0.6;\n    Control.Vref_Red=0.6;\n    \n    if Control.Distance2Master(GreyID)>Control.Platooning_Distance-0.2 && Control.Distance2Master(GreyID)<Control.Platooning_Distance+0.2 && Control.Distance2Master(BlueID)>Control.Platooning_Distance-0.2 && Control.Distance2Master(BlueID)<Control.Platooning_Distance+0.2\n        String='The blue and grey truck are platooning!';\n        MasterID=BlueID;\n    elseif Control.Distance2Master(GreyID)>Control.Platooning_Distance-0.2 && Control.Distance2Master(GreyID)<Control.Platooning_Distance+0.2\n        String='The grey truck is platooning!';\n    elseif Control.Distance2Master(BlueID)>Control.Platooning_Distance-0.2 && Control.Distance2Master(BlueID)<Control.Platooning_Distance+0.2\n        String='The blue truck is platooning!';\n    else\n        String=sprintf('Catching up...\\n');\n    end\n    else\n     MasterID=BlueID;\n    Control.Platooning_Distance=0.3;\n    Control.Vref_Blue=0.6;\n    Control.Vref_Grey=0.6;\n    Control.Vref_Red=0.6;\n    \n    if Control.Distance2Master(GreyID)>Control.Platooning_Distance-0.2 && Control.Distance2Master(GreyID)<Control.Platooning_Distance+0.2 && Control.Distance2Master(RedID)>Control.Platooning_Distance-0.2 && Control.Distance2Master(RedID)<Control.Platooning_Distance+0.2\n        String='The red and grey truck are platooning!';\n    elseif Control.Distance2Master(GreyID)>Control.Platooning_Distance-0.2 && Control.Distance2Master(GreyID)<Control.Platooning_Distance+0.2\n        String='The grey truck is platooning!';\n    elseif Control.Distance2Master(RedID)>Control.Platooning_Distance-0.2 && Control.Distance2Master(RedID)<Control.Platooning_Distance+0.2\n        String='The red truck is platooning!';\n    else\n        String=sprintf('Overtaking...\\n');\n    end\n    end\n\nend"("Control"=w6838, "FirstTime"=w6837, "MasterID"=w6836, "RealSpeed"=w6835, "Positioned"=w6832, "SetMasterID"=w6830) -> ("Control"=w6840:T1, "FirstTime"=w6839:bool, "MasterID"=w6834:i32, "String"=w6833:string, "Positioned"=w6831:bool)  [unwired: 1 in, 1 out]
          "SetMasterID" <- w6834
          n39 = global write "Global.vi" "FirstTime"(w6839) -> ()
          n40 = global write "Global.vi" "Positioned"(w6831) -> ()
          n41 = global write "Global.vi" "SetMasterID"(w6834) -> ()
        }
        frame 8 {
          n42 = mathscript code="String='';\n\nBlueID=1;\nBlackID=2;\nRedID=3;\n\nGreyID=4;\nDarkGreyID=5;\n\n%FirstWPBlue=1;\n%FirstWPBlack=30;\n%FirstWPRed=1;\n%FirstWPGrey=1;\n%FirstWPDarkGrey=1;\n\nControl.Change_to_state_Blue=2;\nControl.Change_to_state_Black=1;\nControl.Change_to_state_Red=2;\nControl.Change_to_state_Grey=2;\nControl.Change_to_state_DarkGrey=1;\n\nControl.With_Trailer_Blue=true;\nControl.With_Trailer_Black=false;\nControl.With_Trailer_Red=true;\nControl.With_Trailer_Grey=true;\nControl.With_Trailer_DarkGrey=false;\n\n\n%Control.Platooning_Distance=2;\n\nif FirstTime\n    if ~Positioned\n            Control.Vref_Red=0.6;\n        if Control.CurrentWP(RedID)<=1\n            String='Positioning the red truck...';\n            Control.Vref_Blue=0;\n            Control.Vref_Grey=0;\n            Control.Vref_Red=0.6;\n        elseif Control.CurrentWP(GreyID)<=1\n            String='Positioning the grey truck...';\n            Control.Vref_Red=0.6;\n            Control.Vref_Blue=0;\n            Control.Vref_Grey=0.6;\n        elseif Control.CurrentWP(BlueID)<=1\n            String='Positioning the blue truck...';\n            Control.Vref_Red=0.6;\n            Control.Vref_Blue=0.6;\n            Control.Vref_Grey=0.6;\n        else\n            Control.Vref_Red=0.6;\n            Control.Vref_Blue=0.6;\n            Control.Vref_Grey=0.6;\n            Positioned=true;\n        end\n    else\n        String='Stabilization Lap.';\n        MasterID=RedID;\n        Control.Distance2Master(BlueID)=Control.Distance2Master(BlueID)-2.7;\n        Control.Platooning_Distance=0.3;\n        Control.Vref_Blue=0.6;\n        Control.Vref_Grey=0.6;\n        Control.Vref_Red=0.6;\n        if Control.CurrentWP(RedID)==1\n            String='#allpositioned';\n            FirstTime=false;\n        end\n    end\nelse\n    \n    if Control.CurrentWP(GreyID)==1\n        LapCounter=LapCounter+1;\n    end\n\n     if LapCounter>5\n        Control.Change_to_state_Grey=3;\n        string='The middle one exited the road. The platoon is remaid trucks are now alone...'\n     end \n    \n    MasterID=RedID;\n    Control.Platooning_Distance=0.3;\n    Control.Vref_Blue=0.6;\n    Control.Vref_Grey=0.6;\n    Control.Vref_Red=0.6;\n    \n    if Control.Distance2Master(GreyID)>Control.Platooning_Distance-0.2 && Control.Distance2Master(GreyID)<Control.Platooning_Distance+0.2 && Control.Distance2Master(BlueID)>Control.Platooning_Distance-0.2 && Control.Distance2Master(BlueID)<Control.Platooning_Distance+0.2\n        String='The blue and grey truck are platooning!';\n    elseif Control.Distance2Master(GreyID)>Control.Platooning_Distance-0.2 && Control.Distance2Master(GreyID)<Control.Platooning_Distance+0.2\n        String='The grey truck is platooning!';\n    elseif Control.Distance2Master(BlueID)>Control.Platooning_Distance-0.2 && Control.Distance2Master(BlueID)<Control.Platooning_Distance+0.2\n        String='The blue truck is platooning!';\n    else\n        String=sprintf('Catching up...\\n');\n    end\n    \nend"("Control"=w8536, "FirstTime"=w8535, "MasterID"=w8534, "RealSpeed"=w8533, "Positioned"=w8530, "LapCounter"=w8528) -> ("Control"=w8538:T1, "FirstTime"=w8537:bool, "MasterID"=w8532:i32, "String"=w8531:string, "Positioned"=w8529:bool, "LapCounter"=w8527:i32)  [unwired: 1 in, 1 out]
          n43 = global write "Global.vi" "SetMasterID"(w8532) -> ()
          n44 = global write "Global.vi" "FirstTime"(w8537) -> ()
          n45 = global write "Global.vi" "Lap Counter"(w8527) -> ()
          n46 = global write "Global.vi" "Positioned"(w8529) -> ()
        }
      }
      "Positioned" <- w18
      "LapCounter" <- w16
    }
    frame 1 {
      n47 = global read "Global.vi" "TL  Inner"() -> (w9903:bool)
      n48 = global read "Global.vi" "TL Outer"() -> (w9904:bool)
      n49 = case shown="4" w9910 {
        tunnel: [w9912 w9924 w11057 w12101 w13187 w14487 w15824] -> w9909
        tunnel: w9908 -> [_ w9922 w11055 w12099 w13185 w14485 w15822]
        tunnel: w9907 -> [w9912 w9920 w11053 w12097 w13183 w14483 w15820]
        tunnel: w9906 -> [_ w9919 w11049 w12095 w13181 w14481 w15818]
        tunnel: w9905 -> [_ w9918 w11050 w12094 w13180 w14480 w15817]
        tunnel: w9904 -> [_ w9917 w11052 w12092 w13177 w14478 w15815]
        tunnel: w9903 -> [_ w9916 w11051 w12093 w13179 w14479 w15816]
        tunnel: ["Manual" ("String") w9913 w11047 w12091 w13178 w14477 w15814] -> w9902
        tunnel: w9901 -> [_ _ w11046 _ _ _ _]
        frame 0, Default {
        }
        frame 1 {
          # "Simple Traffic Lights"
          n50 = mathscript code="String='';\n\n%stop=false;\n\nTrafficLights=[TLOuter,TLInner];\n\nBlackTrajLength=0;\nGreyTrajLength=0;\nBlueTrajLength=0;\n\nBlue=1;\nBlack=2;\nGrey=3;\n\nFirstWP=[2 2 0];\n\ntruck_stop=true;\n\nControl.Change_to_state_Blue=2;\nControl.Change_to_state_Black=1;\n\nControl.With_Trailer_Blue=false;\nControl.With_Trailer_Black=true;\n\nMasterID=0;\n\nif FirstTime\n    \n     % Positioning of the trucks\n\n     TrafficLights=[false,false];\n  \n    if Control.CurrentWP(Black)~=FirstWP(Black)\n        speeds(Blue)=0;\n        if abs(FirstWP(Black)-Control.CurrentWP(Black))>10\n            speeds(Black)=0.5;\n        else\n            speeds(Black)=0.3\n        end\n         String=sprintf('Positioning Black ... Current wp:%g ... First wp:%g ... speed:%.2f',Control.CurrentWP(Black),FirstWP(Black),Control.Vref_Black);\n    elseif Control.CurrentWP(Blue)~=FirstWP(Blue)\n        speeds(Black)=0;\n        if abs(FirstWP(Blue)-Control.CurrentWP(Blue))>10\n            speeds(Blue)=0.5;\n        else\n            speeds(Blue)=0.3\n        end\n        String=sprintf('Positioning Blue ... Current wp:%g ... First wp:%g ... speed:%.2f',Control.CurrentWP(Blue),FirstWP(Blue),Control.Vref_Blue);\n    else\n        speeds=[0  0 0];\n        String='#allpositioned';\n        FirstTime=false;\n    end\n    \nelse\n        \n    %  Traffic Control\n\n    String='Traffic Control';\n\n    speeds=[0.8 0.8 0];\n\n    if ~truck_stop\n\n    if Control.d2TL(Black)<3\n      TrafficLights=[false,true];\n    elseif Control.d2TL(Black)< 13\n      TrafficLights=[false,false];\n    end\n\n\n\n    else\n\n    if Control.d2TL(Blue)<3\n      TrafficLights=[true,false];\n    elseif Control.d2TL(Blue)< 11\n      TrafficLights=[false,false];\n    end\n\n    end\n\n    %if Control.CurrentWP(Black)\n       %stop=true;\n    %end\n\n\nend \n\n Control.Vref_Blue=speeds(Blue);\n Control.Vref_Black=speeds(Black);"("Control"=w9920, "FirstTime"=w9922, "MasterID"=w9919, "RealSpeed"=w9918, "TLOuter"=w9917, "TLInner"=w9916) -> ("Control"=w9924:T1, "TrafficLights"=w9923:bool[], "FirstTime"=w9921:bool, "MasterID"=w9914:i32, "String"=w9913:string)  [unwired: 1 in, 1 out]
          n51 = global write "Global.vi" "FirstTime"(w9921) -> ()
          n52 = Index Array(array=w9923) -> (element #1=w9915:bool, element #2=w9925:bool)  [unwired: 2 in]
          n53 = global write "Global.vi" "SetMasterID"(w9914) -> ()
          n54 = global write "Global.vi" "TL  Inner"(w9925) -> ()
          n55 = global write "Global.vi" "TL Outer"(w9915) -> ()
        }
        frame 2 {
          # "Simple Anti-Platoon"
          n56 = mathscript code="String='';\n\nTrafficLights=[TLOuter,TLInner];\n\nBlue=1;\nBlack=2;\nGrey=4;\n\nspeeds=zeros(length(Control.CurrentWP));\n\nFirstWP=[10 15 0 5];\n\nControl.Change_to_state_Blue=1;\nControl.Change_to_state_Black=1;\nControl.Change_to_state_Grey=1;\n\nControl.With_Trailer_Blue=true;\nControl.With_Trailer_Black=true;\nControl.With_Trailer_Grey=true;\n\nif FirstTime\n\n     MasterID=0\n    \n     TrafficLights=[false,false];\n    \n    if Control.CurrentWP(Black)~=FirstWP(Black)\n        String=sprintf('Positioning Black Truck ... Current wp:%g ... First wp:%g ',Control.CurrentWP(Black),FirstWP(Black));\n        speeds(Black)=0.3;\n    elseif Control.CurrentWP(Blue)~=FirstWP(Blue)\n        String=sprintf('Positioning Blue Truck ... Current wp:%g ... First wp:%g ',Control.CurrentWP(Blue),FirstWP(Blue));\n        speeds(Blue)=0.3;\n    elseif Control.CurrentWP(Grey)~=FirstWP(Grey)\n        String=sprintf('Positioning Grey Truck ... Current wp:%g ... First wp:%g ',Control.CurrentWP(Grey),FirstWP(Grey));\n        speeds(Grey)=0.3;\n    else\n        FirstTime=false;\n        Positioned=true;\n        String='#allpositioned';\n    end\n    \nelse\n\n    String='Platooning';\n\n    TrafficLights=[false,false];\n\n    time_gap=3;\n\n     Control.Platooning_Distance=RealSpeed(Grey)*time_gap;\n\n     MasterID=Black;\n   \n    speeds(Black)=0.6;\n    speeds(Blue)=0.6;\n    speeds(Grey)=0.6;\n\nend\n\n Control.Vref_Blue=speeds(Blue);\n Control.Vref_Black=speeds(Black);\n Control.Vref_Grey=speeds(Grey);"("Control"=w11053, "FirstTime"=w11055, "TLOuter"=w11052, "TLInner"=w11051, "RealSpeed"=w11050, "MasterID"=w11049, "Positioned"=w11046) -> ("Control"=w11057:T1, "TrafficLights"=w11056:bool[], "FirstTime"=w11054:bool, "MasterID"=w11048:i32, "String"=w11047:string, "Positioned"=w11045:bool)  [unwired: 1 in, 1 out]
          n57 = Index Array(array=w11056) -> (element #1=w11058:bool, element #2=w11059:bool)  [unwired: 2 in]
          n58 = global write "Global.vi" "SetMasterID"(w11048) -> ()
          n59 = global write "Global.vi" "Positioned"(w11045) -> ()
          n60 = global write "Global.vi" "FirstTime"(w11054) -> ()
          n61 = global write "Global.vi" "TL Outer"(w11058) -> ()
          n62 = global write "Global.vi" "TL  Inner"(w11059) -> ()
        }
        frame 3 {
          # "Mixture"
          n63 = mathscript code="TrafficLights=[false,false];\n\nString='';\n\nTrafficLights=[TLOuter,TLInner];\n\nBlue=1;\nBlack=2;\nGrey=4;\n\nspeeds=zeros(length(Control.CurrentWP));\n\nFirstWP=[5 10 0 50];\n\nControl.Change_to_state_Blue=2;\nControl.Change_to_state_Black=2;\nControl.Change_to_state_Grey=1;\n\n\nControl.With_Trailer_Blue=true;\n% Carro\nControl.With_Trailer_Black=false;\nControl.With_Trailer_Grey=true;\n\nMasterID=0\n\nif FirstTime\n\n     MasterID=0\n    \n     TrafficLights=[false,false];\n    \n    if Control.CurrentWP(Black)~=FirstWP(Black)\n        String=sprintf('Positioning Black Truck ... Current wp:%g ... First wp:%g ',Control.CurrentWP(Black),FirstWP(Black));\n        speeds(Black)=0.3;\n    elseif Control.CurrentWP(Blue)~=FirstWP(Blue)\n        String=sprintf('Positioning Blue Truck ... Current wp:%g ... First wp:%g ',Control.CurrentWP(Blue),FirstWP(Blue));\n        speeds(Blue)=0.3;\n    elseif Control.CurrentWP(Grey)~=FirstWP(Grey)\n        String=sprintf('Positioning Grey Truck ... Current wp:%g ... First wp:%g ',Control.CurrentWP(Grey),FirstWP(Grey));\n        speeds(Grey)=0.3;\n    else\n        String='#allpositioned';\n        FirstTime=false;\n    end\n    \nelse\n\n     MasterID=Black\n\n     speeds=[0.6 0.6 0 0.6];\n\n    if Control.d2TL(Grey)<3\n      speeds(Blue)=0.3;\n      TrafficLights=[false,true];\n    elseif Control.d2TL(Grey)<13\n      speeds(Blue)=0.6;\n      TrafficLights=[false,false];\n    end\n\nend\n\n Control.Vref_Blue=speeds(Blue);\n Control.Vref_Black=speeds(Black);\n Control.Vref_Grey=speeds(Grey);"("Control"=w12097, "FirstTime"=w12099, "MasterID"=w12095, "RealSpeed"=w12094, "TLOuter"=w12092, "TLInner"=w12093) -> ("Control"=w12101:T1, "TrafficLights"=w12100:bool[], "FirstTime"=w12098:bool, "MasterID"=w12096:i32, "String"=w12091:string)  [unwired: 1 in, 1 out]
          n64 = global write "Global.vi" "FirstTime"(w12098) -> ()
          n65 = global write "Global.vi" "SetMasterID"(w12096) -> ()
          n66 = Index Array(array=w12100) -> (element #1=w12102:bool, element #2=w12103:bool)  [unwired: 2 in]
          n67 = global write "Global.vi" "TL Outer"(w12102) -> ()
          n68 = global write "Global.vi" "TL  Inner"(w12103) -> ()
        }
        frame 4 {
          # "Time Decision"
          n69 = mathscript code="TrafficLights=[false,false];\n\nString='';\n\nTrafficLights=[TLOuter,TLInner];\n\nBlue=1;\nBlack=2;\nGrey=4;\n\nFirstWP=[0 1 0 1];\n\nChangeTraffic=false;\n\nspeeds=zeros(length(Control.CurrentWP));\n\nControl.Change_to_state_Blue=2;\nControl.Change_to_state_Black=2;\nControl.Change_to_state_Grey=1;\n\nControl.With_Trailer_Blue=true;\nControl.With_Trailer_Black=false;\nControl.With_Trailer_Grey=true;\n\nMasterID=0\n\n\nif FirstTime\n\n     MasterID=0\n    \n     TrafficLights=[false,false];\n    \n    if Control.CurrentWP(Black)~=FirstWP(Black)\n        String=sprintf('Positioning Black Truck ... Current wp:%g ... First wp:%g ',Control.CurrentWP(Black),FirstWP(Black));\n        speeds(Black)=0.3;\n    elseif Control.CurrentWP(Blue)~=FirstWP(Blue)\n        String=sprintf('Positioning Blue Truck ... Current wp:%g ... First wp:%g ',Control.CurrentWP(Blue),FirstWP(Blue));\n         speeds(Blue)=0.3;\n    elseif Control.CurrentWP(Grey)~=FirstWP(Grey)\n        String=sprintf('Positioning Grey Truck ... Current wp:%g ... First wp:%g ',Control.CurrentWP(Grey),FirstWP(Grey));\n         speeds(Grey)=0.3;\n    else\n        String='#allpositioned';\n        FirstTime=false;\n    end\n    \nelse\n\n    speeds=[0.6 0.6 0 0.6];\n\n     \n\n     time2TL=Control.d2TL./RealSpeed;\n\n\n\n\n     %[times closest_truck]=sort(time2TL);\n\n\n     %truck=closest_truck(1);\n    %if TrafficLights(Control.CurrentState(closest_truck(1)))==true\n      %truck=closest_truck(1);\n    %elseif TrafficLights(Control.CurrentState(closest_truck(2)))==true\n      %truck=closest_truck(2);\n    %end\n\n    %if TrafficLights(1)==true  || TrafficLights(2)==true\n       %   ChangeTraffic=true;\n    %end\n\n    %String=sprintf('none %g  ChangeTraffic %g',closest_truck(2),ChangeTraffic);\n\n    %if  Control.d2TL(closest_truck(1))<3 &&  ~ChangeTraffic && Control.d2TL(closest_truck(2))<6\n        %TrafficLights(Control.CurrentState(closest_truck(1)))=false;\n        %TrafficLights(rem(Control.CurrentState(closest_truck(1)),2)+1)=true;\n           %String=sprintf('change closest %g  second %g ChangeTraffic %g t1 %g t2  %g ',closest_truck(1),closest_truck(2),ChangeTraffic,TrafficLights(1),TrafficLights(2));\n          %speeds(closest_truck(2)) =Control.d2TL(closest_truck(2))/(time2TL(closest_truck(2))+2);    \n          \n          %ChangeTraffic=true;\n\n        %if speeds(closest_truck(2))<0.3\n           % speeds(closest_truck(2))=0.3;\n        %end\n\n     %elseif  Control.d2TL(closest_truck(2))< 12 &&  ChangeTraffic\n         %speeds(closest_truck(2)) =0.8;\n        %TrafficLights=[false,false];\n          %String=sprintf('clear %g ',truck);\n     %end\n\n\n     if  Control.d2TL(Black)<4 ||  Control.d2TL(Black)>12\n         TrafficLights(Control.CurrentState(Grey))=true;\n         speeds(Grey) =Control.d2TL(Grey)/(time2TL(Grey)+2);       \n\n          if speeds(Grey)<0.3\n              speeds(Grey)=0.3;\n          end\n\n\n      elseif Control.d2TL(Black)>4 &&  Control.d2TL(Black)<12\n          TrafficLights(Control.CurrentState(Grey))=false;\n           speeds(Grey)=0.6;\n     end\n\n\n\nend\n\n Control.Vref_Blue=speeds(Blue);\n Control.Vref_Black=speeds(Black);\n Control.Vref_Grey=speeds(Grey);"("Control"=w13183, "FirstTime"=w13185, "MasterID"=w13181, "RealSpeed"=w13180, "TLOuter"=w13177, "TLInner"=w13179) -> ("Control"=w13187:T1, "TrafficLights"=w13186:bool[], "FirstTime"=w13184:bool, "MasterID"=w13182:i32, "String"=w13178:string)  [unwired: 1 in, 1 out]
          n70 = global write "Global.vi" "FirstTime"(w13184) -> ()
          n71 = global write "Global.vi" "SetMasterID"(w13182) -> ()
          n72 = Index Array(array=w13186) -> (element #1=w13188:bool, element #2=w13189:bool)  [unwired: 2 in]
          n73 = global write "Global.vi" "TL Outer"(w13188) -> ()
          n74 = global write "Global.vi" "TL  Inner"(w13189) -> ()
        }
        frame 5 {
          # "Timed Control with Platoon"
          n75 = mathscript code="TrafficLights=[false,false];\n\nString='';\n\nTrafficLights=[TLOuter,TLInner];\n\nBlue=1;\nBlack=2;\nRed=3;\n\nFirstWP=[20 1 20];\n\nControl.Change_to_state_Blue=2;\nControl.Change_to_state_Black=1;\nControl.Change_to_state_Red=1;\n\nPlatoon=[Black Red];\n\nControl.With_Trailer_Blue=true;\nControl.With_Trailer_Black=true;\nControl.With_Trailer_Red=true;\n\nMasterID=0\n\nif FirstTime\n    \n    MasterID=0;\n    \n    TrafficLights=[false,false];\n    \n    if Control.CurrentWP(Black)~=FirstWP(Black)\n        String=sprintf('Positioning Black Truck ... Current wp:%g ... First wp:%g ',Control.CurrentWP(Black),FirstWP(Black));\n        speeds=[0 0.3 0];\n    elseif Control.CurrentWP(Blue)~=FirstWP(Blue)\n        String=sprintf('Positioning Blue Truck ... Current wp:%g ... First wp:%g ',Control.CurrentWP(Blue),FirstWP(Blue));\n        speeds=[0.3 0 0];\n    elseif Control.CurrentWP(Red)~=FirstWP(Red)\n        String=sprintf('Positioning Red Truck ... Current wp:%g ... First wp:%g ',Control.CurrentWP(Red),FirstWP(Red));\n        speeds=[0 0 0.3]\n    else\n        speeds=[0 0 0]\n        FirstTime=false;\n    end\n    \nelse\n    \n    MasterID=Black,\n    \n    speeds=[0.8 0.8 0.8];\n    \n    time2TL=Control.d2TL./RealSpeed;\n    \n    [times closest_truck]=sort(time2TL);\n    \n    i=1;\n    \n    closest_final=[];\n    while i<=length(speeds)\n        if ~isempty(find(Platoon,closest_truck(i)))\n            if closest_truck(i)==Platoon(length(Platoon))\n                closest_final=[closest_final closest_truck(i)];\n            end\n        else\n            closest_final=[closest_final closest_truck(i)];\n        end\n        i=i+1\n    end\n    \n    closest_truck=closest_final;\n    \n    if  Control.d2TL(closest_truck(1))<3\n        TrafficLights(Control.CurrentState(closest_truck(1)))=false;\n        TrafficLights(rem(Control.CurrentState(closest_truck(1))+1,1))=true;\n        speeds(closest_truck(2)) =Control.d2TL(closest_truck(1))/(time2TL(1)+2);\n        \n    else\n        speeds(closest_truck(2)) =0.8;\n        TrafficLights=[false,false];\n    end\n    \nend\n\nControl.Vref_Blue=speeds(Blue);\nControl.Vref_Black=speeds(Black);\nControl.Vref_Red=speeds(Red);"("Control"=w14483, "FirstTime"=w14485, "MasterID"=w14481, "RealSpeed"=w14480, "TLOuter"=w14478, "TLInner"=w14479) -> ("Control"=w14487:T1, "TrafficLights"=w14486:bool[], "FirstTime"=w14484:bool, "MasterID"=w14482:i32, "String"=w14477:string)  [unwired: 1 in, 1 out]
          n76 = global write "Global.vi" "FirstTime"(w14484) -> ()
          n77 = global write "Global.vi" "SetMasterID"(w14482) -> ()
          n78 = Index Array(array=w14486) -> (element #1=w14488:bool, element #2=w14489:bool)  [unwired: 2 in]
          n79 = global write "Global.vi" "TL Outer"(w14488) -> ()
          n80 = global write "Global.vi" "TL  Inner"(w14489) -> ()
        }
        frame 6 {
          n81 = mathscript code="String='';\n\nTrafficLights=[TLOuter,TLInner];\n\nBlue=1;\nBlack=2;\nGrey=4;\n\nspeeds=zeros(length(Control.CurrentWP));\n\nFirstWP=[0 15 0 5];\n\nControl.Change_to_state_Blue=2;\nControl.Change_to_state_Black=1;\nControl.Change_to_state_Grey=1;\n\nControl.With_Trailer_Blue=true;\nControl.With_Trailer_Black=true;\nControl.With_Trailer_Grey=true;\n\nif FirstTime\n\n     MasterID=0\n    \n     TrafficLights=[false,false];\n    \n    if Control.CurrentWP(Black)~=FirstWP(Black)\n        String=sprintf('Positioning Black Truck ... Current wp:%g ... First wp:%g ',Control.CurrentWP(Black),FirstWP(Black));\n        speeds(Black)=0.3;\n    elseif Control.CurrentWP(Blue)~=FirstWP(Blue)\n        String=sprintf('Positioning Blue Truck ... Current wp:%g ... First wp:%g ',Control.CurrentWP(Blue),FirstWP(Blue));\n        speeds(Blue)=0.3;\n    elseif Control.CurrentWP(Grey)~=FirstWP(Grey)\n        String=sprintf('Positioning Grey Truck ... Current wp:%g ... First wp:%g ',Control.CurrentWP(Grey),FirstWP(Grey));\n        speeds(Grey)=0.3;\n    else\n        FirstTime=false;\n        Positioned=true;\n        String='#allpositioned';\n    end\n    \nelse\n\n    String='Platooning';\n\n    TrafficLights=[false,false];\n\n     time_gap=10;\n\n     MasterID=Black;\n   \n    speeds(Black)=0.9;\n\n     Control.Platooning_Distance=RealSpeed(Grey)*time_gap;\n\nend\n\n Control.Vref_Blue=speeds(Blue);\n Control.Vref_Black=speeds(Black);\n Control.Vref_Grey=speeds(Grey);"("Control"=w15820, "FirstTime"=w15822, "MasterID"=w15818, "RealSpeed"=w15817, "TLOuter"=w15815, "TLInner"=w15816) -> ("Control"=w15824:T1, "TrafficLights"=w15823:bool[], "FirstTime"=w15821:bool, "MasterID"=w15819:i32, "String"=w15814:string)  [unwired: 1 in, 1 out]
          n82 = global write "Global.vi" "FirstTime"(w15821) -> ()
          n83 = global write "Global.vi" "SetMasterID"(w15819) -> ()
          n84 = Index Array(array=w15823) -> (element #1=w15825:bool, element #2=w15826:bool)  [unwired: 2 in]
          n85 = global write "Global.vi" "TL Outer"(w15825) -> ()
          n86 = global write "Global.vi" "TL  Inner"(w15826) -> ()
        }
      }
    }
  }
  "String" <- w5
  "Control Out" <- w3
